vi "Configuration.vi"(0 "App Path":path=path "C:/Users/gtetil/Documents/Projects/DAQ Rack/Source", 5 "Config Path":path, 7 "Cal Base Path":path) -> (6 "Config Path OUT":path)   [LabVIEW 2019]
uses:
  Type Defs and Controls/Sensor List Cluster.ctl
  Type Defs and Controls/Channel Config Screen.ctl
  Type Defs and Controls/Log File Type.ctl
  Type Defs and Controls/Registered System.ctl
  Type Defs and Controls/System Type.ctl
  Type Defs and Controls/Sensor Config.ctl
  Type Defs and Controls/DAQ Settings.ctl
  Type Defs and Controls/Trigger Stop Method.ctl
  Type Defs and Controls/Channel Config.ctl
  Type Defs and Controls/Header.ctl
  Type Defs and Controls/Graph Settings Type Def.ctl
  Type Defs and Controls/Test Limits.ctl
  Type Defs and Controls/All Part Info.ctl
  Type Defs and Controls/Part Info.ctl
  <vilib>/Utility/config.llb/Write Key (Path).vi
  <vilib>/Utility/config.llb/NI_LVConfig.lvlib
panel:
  in  "TCP Stream Ref":refnum<vi>
  in  "System":T1={"System Type"=enum."DAQ Cart", "Serial Number"=0, "ID"="", "Cal File?"=FALSE}
  in  "Log File Type":T3
  in  "Part Config":bool
  in  "Limit:":dbl caption="Mb"
  in  "Hide Trig Ch":bool
  in  "Hide Trig Val":bool
  in  "Hide Trig Samples":bool
  in  "Hide Trig Stop":bool
  in  "Hide Trig Int":bool
  in  "Hide Pretrig Smpls":bool
  in  "Save Mode":T4(ring)
  in  "Sample Min":bool
  in  "Sample Sec":bool
  out "Changes Latch":bool
  out "Changes?":bool
  in  "Revert":bool
  out "Config Name":string
  in  "debug":bool
  in  "Delete Sensor":bool
  in  "Add Sensor":bool
  in  "Save As":bool
  in  "Save":bool
  in  "Open":bool
  in  "Calling VI Ref":refnum<vi>
  in  "Auto Save":bool=TRUE
  in  "Trigger Stop Method":T5(ring)
  in  "Hours":bool
  in  "Minutes":bool
  in  "Trigger Type":T6(ring)
  in  "Header Table":string[][](table)=[[""], [""], [""], [""], [""], [""]]
  in  "Sensors":T7=[{"Channel"="9221_AI-00", "Description"="", "Acquire"=FALSE, "Sensor"="None Selected", "Chg Sensor"=FALSE, "Cal Date"="---------", "Offset"=0.0, "Span"=0.0, "Cal"=FALSE, "Test Limits"=FALSE, "Type"="0-60 VDC", "Data Index"=0}, {"Channel"="9221_AI-01", "Description"="", "Acquire"=FALSE, "Sensor"="None Selected", "Chg Sensor"=FALSE, "Cal Date"="---------", "Offset"=0.0, "Span"=0.0, "Cal"=FALSE, "Test Limits"=FALSE, "Type"="0-60 VDC", "Data Index"=1}, {"Channel"="9221_AI-02", "Description"="", "Acquire"=FALSE, "Sensor"="None Selected", "Chg Sensor"=FALSE, "Cal Date"="---------", "Offset"=0.0, "Span"=0.0, "Cal"=FALSE, "Test Limits"=FALSE, "Type"="0-60 VDC", "Data Index"=2}, {"Channel"="9221_AI-03", "Description"="", "Acquire"=FALSE, "Sensor"="None Selected", "Chg Sensor"=FALSE, "Cal Date"="---------", "Offset"=0.0, "Span"=0.0, "Cal"=FALSE, "Test Limits"=FALSE, "Type"="0-60 VDC", "Data Index"=3}, {"Channel"="9221_AI-04", "Description"="", "Acquire"=FALSE, "Sensor"="None Selected", "Chg Sensor"=FALSE, "Cal Date"="---------", "Offset"=0.0, "Span"=0.0, "Cal"=FALSE, "Test Limits"=FALSE, "Type"="0-60 VDC", "Data Index"=4}, {"Channel"="9221_AI-05", "Description"="", "Acquire"=FALSE, "Sensor"="None Selected", "Chg Sensor"=FALSE, "Cal Date"="---------", "Offset"=0.0, "Span"=0.0, "Cal"=FALSE, "Test Limits"=FALSE, "Type"="0-60 VDC", "Data Index"=5}, {"Channel"="9221_AI-06", "Description"="", "Acquire"=FALSE, "Sensor"="None Selected", "Chg Sensor"=FALSE, "Cal Date"="---------", "Offset"=0.0, "Span"=0.0, "Cal"=FALSE, "Test Limits"=FALSE, "Type"="0-60 VDC", "Data Index"=6}, {"Channel"="9221_AI-07", "Description"="", "Acquire"=FALSE, "Sensor"="None Selected", "Chg Sensor"=FALSE, "Cal Date"="---------", "Offset"=0.0, "Span"=0.0, "Cal"=FALSE, "Test Limits"=FALSE, "Type"="0-60 VDC", "Data Index"=7}, {"Channel"="9205_AI-00", "Description"="", "Acquire"=FALSE, "Sensor"="None Selected", "Chg Sensor"=FALSE, "Cal Date"="---------", "Offset"=0.0, "Span"=0.0, "Cal"=FALSE, "Test Limits"=FALSE, "Type"="0-10 VDC", "Data Index"=8}, {"Channel"="9205_AI-01", "Description"="", "Acquire"=FALSE, "Sensor"="None Selected", "Chg Sensor"=FALSE, "Cal Date"="---------", "Offset"=0.0, "Span"=0.0, "Cal"=FALSE, "Test Limits"=FALSE, "Type"="0-10 VDC", "Data Index"=9}, {"Channel"="9205_AI-02", "Description"="", "Acquire"=FALSE, "Sensor"="None Selected", "Chg Sensor"=FALSE, "Cal Date"="---------", "Offset"=0.0, "Span"=0.0, "Cal"=FALSE, "Test Limits"=FALSE, "Type"="0-10 VDC", "Data Index"=10}, {"Channel"="9205_AI-03", "Description"="", "Acquire"=FALSE, "Sensor"="None Selected", "Chg Sensor"=FALSE, "Cal Date"="---------", "Offset"=0.0, "Span"=0.0, "Cal"=FALSE, "Test Limits"=FALSE, "Type"="0-10 VDC", "Data Index"=11}, {"Channel"="9205_AI-04", "Description"="", "Acquire"=FALSE, "Sensor"="None Selected", "Chg Sensor"=FALSE, "Cal Date"="---------", "Offset"=0.0, "Span"=0.0, "Cal"=FALSE, "Test Limits"=FALSE, "Type"="0-10 VDC", "Data Index"=12}, {"Channel"="9205_AI-05", "Description"="", "Acquire"=FALSE, "Sensor"="None Selected", "Chg Sensor"=FALSE, "Cal Date"="---------", "Offset"=0.0, "Span"=0.0, "Cal"=FALSE, "Test Limits"=FALSE, "Type"="0-10 VDC", "Data Index"=13}, {"Channel"="9205_AI-06", "Description"="", "Acquire"=FALSE, "Sensor"="None Selected", "Chg Sensor"=FALSE, "Cal Date"="---------", "Offset"=0.0, "Span"=0.0, "Cal"=FALSE, "Test Limits"=FALSE, "Type"="0-10 VDC", "Data Index"=14}, {"Channel"="9205_AI-07", "Description"="", "Acquire"=FALSE, "Sensor"="None Selected", "Chg Sensor"=FALSE, "Cal Date"="---------", "Offset"=0.0, "Span"=0.0, "Cal"=FALSE, "Test Limits"=FALSE, "Type"="0-10 VDC", "Data Index"=15}, {"Channel"="9208_AI-00", "Description"="", "Acquire"=FALSE, "Sensor"="None Selected", "Chg Sensor"=FALSE, "Cal Date"="---------", "Offset"=0.0, "Span"=0.0, "Cal"=FALSE, "Test Limits"=FALSE, "Type"="0-20 mA", "Data Index"=16}, {"Channel"="9208_AI-01", "Description"="", "Acquire"=FALSE, "Sensor"="None Selected", "Chg Sensor"=FALSE, "Cal Date"="---------", "Offset"=0.0, "Span"=0.0, "Cal"=FALSE, "Test Limits"=FALSE, "Type"="0-20 mA", "Data Index"=17}, {"Channel"="9208_AI-02", "Description"="", "Acquire"=FALSE, "Sensor"="None Selected", "Chg Sensor"=FALSE, "Cal Date"="---------", "Offset"=0.0, "Span"=0.0, "Cal"=FALSE, "Test Limits"=FALSE, "Type"="0-20 mA", "Data Index"=18}, {"Channel"="9208_AI-03", "Description"="", "Acquire"=FALSE, "Sensor"="None Selected", "Chg Sensor"=FALSE, "Cal Date"="---------", "Offset"=0.0, "Span"=0.0, "Cal"=FALSE, "Test Limits"=FALSE, "Type"="0-20 mA", "Data Index"=19}, {"Channel"="9208_AI-04", "Description"="", "Acquire"=FALSE, "Sensor"="None Selected", "Chg Sensor"=FALSE, "Cal Date"="---------", "Offset"=0.0, "Span"=0.0, "Cal"=FALSE, "Test Limits"=FALSE, "Type"="0-20 mA", "Data Index"=20}, {"Channel"="9208_AI-05", "Description"="", "Acquire"=FALSE, "Sensor"="None Selected", "Chg Sensor"=FALSE, "Cal Date"="---------", "Offset"=0.0, "Span"=0.0, "Cal"=FALSE, "Test Limits"=FALSE, "Type"="0-20 mA", "Data Index"=21}, {"Channel"="9208_AI-06", "Description"="", "Acquire"=FALSE, "Sensor"="None Selected", "Chg Sensor"=FALSE, "Cal Date"="---------", "Offset"=0.0, "Span"=0.0, "Cal"=FALSE, "Test Limits"=FALSE, "Type"="0-20 mA", "Data Index"=22}, {"Channel"="9208_AI-07", "Description"="", "Acquire"=FALSE, "Sensor"="None Selected", "Chg Sensor"=FALSE, "Cal Date"="---------", "Offset"=0.0, "Span"=0.0, "Cal"=FALSE, "Test Limits"=FALSE, "Type"="0-20 mA", "Data Index"=23}, {"Channel"="9211_TC-00", "Description"="", "Acquire"=FALSE, "Sensor"="None Selected", "Chg Sensor"=FALSE, "Cal Date"="---------", "Offset"=0.0, "Span"=0.0, "Cal"=FALSE, "Test Limits"=FALSE, "Type"="T-Type", "Data Index"=24}, {"Channel"="9211_TC-01", "Description"="", "Acquire"=FALSE, "Sensor"="None Selected", "Chg Sensor"=FALSE, "Cal Date"="---------", "Offset"=0.0, "Span"=0.0, "Cal"=FALSE, "Test Limits"=FALSE, "Type"="T-Type", "Data Index"=25}, {"Channel"="9211_TC-02", "Description"="", "Acquire"=FALSE, "Sensor"="None Selected", "Chg Sensor"=FALSE, "Cal Date"="---------", "Offset"=0.0, "Span"=0.0, "Cal"=FALSE, "Test Limits"=FALSE, "Type"="T-Type", "Data Index"=26}, {"Channel"="9211_TC-03", "Description"="", "Acquire"=FALSE, "Sensor"="None Selected", "Chg Sensor"=FALSE, "Cal Date"="---------", "Offset"=0.0, "Span"=0.0, "Cal"=FALSE, "Test Limits"=FALSE, "Type"="T-Type", "Data Index"=27}]
  in  "DAQ Table":string[][](table)=[[""], ["AI-00"], ["0.000"], ["0"], ["0"], ["0.000"], [""], ["100"]]
  # "samples /"
  # "Channel"
  # "Type"
  # "Acquire"
  # "Name"
  # "Sensor"
  # "Cal Date"
  # "Zero"
  # "Span"
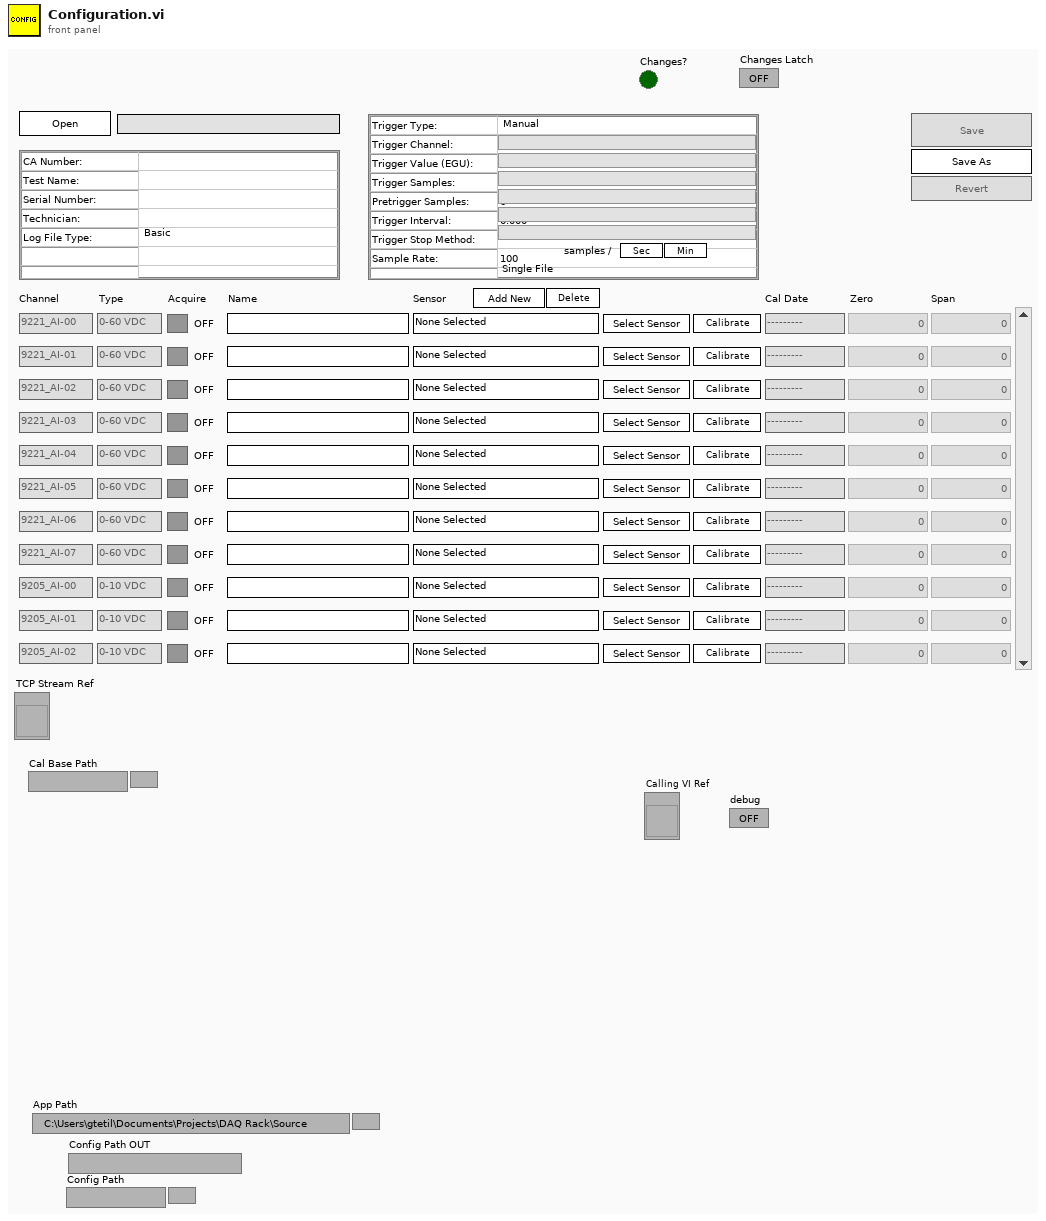
[diagram p1: front panel]
types:
  T1 = typedef "Registered System.ctl" = cluster{"System Type":T2, "Serial Number":u32, "ID":string, "Cal File?":bool}
  T2 = typedef "System Type.ctl" = enum16{"DAQ Rack", "DAQ Cart", "nx-5000", "unknown", "open"}
  T3 = typedef "Log File Type.ctl" = enum16{"Basic", "RTS"}
  T4 = enum16{"Single File", "Segmented Files", "New File at Midnight"}
  T5 = enum16{"Use Samples Value to Stop Trigger", "Use Threshold to Stop Trigger"}
  T6 = enum16{"Manual", "Timed", "Analog Rising", "Analog Falling"}
  T7 = typedef "Sensor List Cluster.ctl" = T8[]
  T8 = typedef "Channel Config Screen.ctl" = cluster{"Channel":string, "Description":string, "Acquire":bool, "Sensor":string, "Chg Sensor":bool, "Cal Date":string, "Offset":dbl, "Span":dbl, "Cal":bool, "Test Limits":bool, "Type":string, "Data Index":u32}
  T9 = typedef "Sensor Config.ctl" = cluster{"DAQ Settings":T10, "Channels":T12[], "Header":T13, "Graph Settings":T14, "Test Limits":T15[], "All Type Info":T16, "Save Mode":enum16{"Single File", "Segmented Files", "New File at Midnight"}}
  T10 = typedef "DAQ Settings.ctl" = cluster{"Trigger Type":enum16{"Manual", "Timed", "Analog Rising", "Analog Falling"}, "Trigger Samples":i32, "Pretrigger Samples":i32, "Trigger Interval":dbl, "Time Units":bool, "Auto Save":bool, "Sample Rate":dbl, "Select Analog":bool, "Trigger Value":dbl, "Trigger Stop Method":T11, "Rate Sec/Min":bool, "Save Mode":enum16{"Single File", "Segmented Files", "New File at Midnight"}, "File Size Limit":dbl, "Log File Type":T3, "Trigger Data Index":u32}
  T11 = typedef "Trigger Stop Method.ctl" = enum16{"Use Samples Value to Stop Trigger", "Use Threshold to Stop Trigger"}
  T12 = typedef "Channel Config.ctl" = cluster{"Channel":string, "Type":string, "Acquire":bool, "Name":string, "Sensor":string, "Data Index":u32}
  T13 = typedef "Header.ctl" = cluster{"TA Number":string, "Test Name":string, "Serial Number":string, "Technician":string}
  T14 = typedef "Graph Settings Type Def.ctl" = cluster{"Graph Labels":string[], u8[], i16[], u32[], u8[], u8[], u8[], u32[], u8[], u8[], u8[], dbl[], dbl[], "Graph Toggles":bool[], "Axis Toggles":bool[], "Graph Range":enum16{"1", "2", "3", "4", "5", "10", "15", "30", "60"}}
  T15 = typedef "Test Limits.ctl" = cluster{"Channel Acquired?":bool, "RMS?":bool, "Pk-Pk":bool, "Frequency":bool, "EU High Limit 1":dbl, "EU Low Limit 1":dbl, "EU High Limit 2":dbl, "EU Low Limit 2":dbl, "RMS High Limit":dbl, "RMS Low Limit":dbl, "Pk-Pk High Limit ":dbl, "Pk-Pk Low Limit":dbl, "Frequency High Limit":dbl, "Frequency Low Limit":dbl}
  T16 = typedef "All Part Info.ctl" = cluster{"Type Name":string, "Type Signal Names":string[], "# Signals":i32, "# Parts":i32, "Part Info":T17[]}[]
  T17 = typedef "Part Info.ctl" = cluster{"Part Number":string, "Channel Indexes":u16[], "Enabled?":bool}
  T18 = cluster{"Sensor Name":string, "Sensor Info":cluster{"Manufacturer":string, "Model":string, "Serial Number":string}, "Last Cal Info":cluster{"Last Calibration Date":dbl, "Calibrator":string, "Cal Duration":i32}, "Voltage Range":cluster{"High Limit":dbl, "Low Limit":dbl}, "EGU Range":cluster{"High Limit":dbl, "Low Limit":dbl}, "Units":string, "Calibration Type":enum16{"Calibrate Analog", "Compare Analog Calibration"}, "EGU List":dbl[], "Voltage List":dbl[], "Coefficients":dbl[], "Order":i32, "Algorithm":enum32{"SVD", "Givens", "Givens2", "Householder", "LU Decomposition", "Cholesky"}, "Max Error % of Full Scale":dbl, "Max Mean Squared Error":dbl, "Use Error %":bool, "Use MSE":bool, "Allow Manual Entry":bool, "Max Stability Error":dbl, "Max Error % of Reading":dbl, "Use Error % of Reading":bool}[]
  T19 = cluster{"Config Path":path, "Channel Select":i32, "Channel Display":T7, "App Path":path, "Config":T9, "Sensors":cluster{"Sensor Name":string, "Sensor Info":cluster{"Manufacturer":string, "Model":string, "Serial Number":string}, "Last Cal Info":cluster{"Last Calibration Date":dbl, "Calibrator":string, "Cal Duration":i32}, "Voltage Range":cluster{"High Limit":dbl, "Low Limit":dbl}, "EGU Range":cluster{"High Limit":dbl, "Low Limit":dbl}, "Units":string, "Calibration Type":enum16{"Calibrate Analog", "Compare Analog Calibration"}, "EGU List":dbl[], "Voltage List":dbl[], "Coefficients":dbl[], "Order":i32, "Algorithm":enum32{"SVD", "Givens", "Givens2", "Householder", "LU Decomposition", "Cholesky"}, "Max Error % of Full Scale":dbl, "Max Mean Squared Error":dbl, "Use Error %":bool, "Use MSE":bool, "Allow Manual Entry":bool, "Max Stability Error":dbl, "Max Error % of Reading":dbl, "Use Error % of Reading":bool}[], "Config Saved":T9, "config start path":path, "Cal Base Path":path, "Calling VI Ref":refnum<vi>, "debug":bool, "Changes?":bool, "Revert":bool, "DAQ Running":bool, "System":T1, "Load Prompt":bool, "App Config Path":path, "TCP Stream Ref":refnum<vi>}
  T20 = enum32{"Bad", "Idle", "Run top level", "Running"}
  T21 = enum8{"Enabled", "Disabled", "Disabled and Grayed Out"}
  T22 = typedef "eventvkey.ctl" = enum16{"ASCII", "Enter", "Return", "Shift", "Ctrl", "Alt", "Cmd", "Opt", "Caps", "NumLock", "Clear", "Break", "Up", "Down", "Left", "Right", "Insert", "Delete", "Home", "End", "PageUp", "PageDown", "Escape", "Help", "Pause", "ScrollLock", "F1", "F2", "F3", "F4", "F5", "F6", "F7", "F8", "F9", "F10", "F11", "F12", "F13", "F14", "F15", "F16", "F17", "F18", "F19", "F20", "F21", "F22", "F23", "F24", "Play", "VolumeUp", "VolumeDown", "Mute", "Two Byte Char"}
  T23 = typedef "LVRowAndColumnTypeDef.ctl" = cluster{"Row":i32, "Column":i32}
  T24 = cluster{"Header Table[0]":string, "Header Table[1]":string, "Header Table[2]":string, "Header Table[3]":string}
  T25 = typedef "LVPoint32TypeDef.ctl" = cluster{"Horizontal":i32, "Vertical":i32}
  T26 = cluster{"Sensor Name":string, "Sensor Info":cluster{"Manufacturer":string, "Model":string, "Serial Number":string}, "Last Cal Info":cluster{"Last Calibration Date":dbl, "Calibrator":string, "Cal Duration":i32}, "Voltage Range":cluster{"High Limit":dbl, "Low Limit":dbl}, "EGU Range":cluster{"High Limit":dbl, "Low Limit":dbl}, "Units":string, "Calibration Type":enum16{"Calibrate Analog", "Compare Analog Calibration"}, "EGU List":dbl[], "Voltage List":dbl[], "Coefficients":dbl[], "Order":i32, "Algorithm":enum32{"SVD", "Givens", "Givens2", "Householder", "LU Decomposition", "Cholesky"}, "Max Error % of Full Scale":dbl, "Max Mean Squared Error":dbl, "Use Error %":bool, "Use MSE":bool, "Allow Manual Entry":bool, "Max Stability Error":dbl, "Max Error % of Reading":dbl, "Use Error % of Reading":bool}
  T27 = typedef "NI_LVConfig.lvlib/Config Data RefNum.ctl" = refnum<k1>
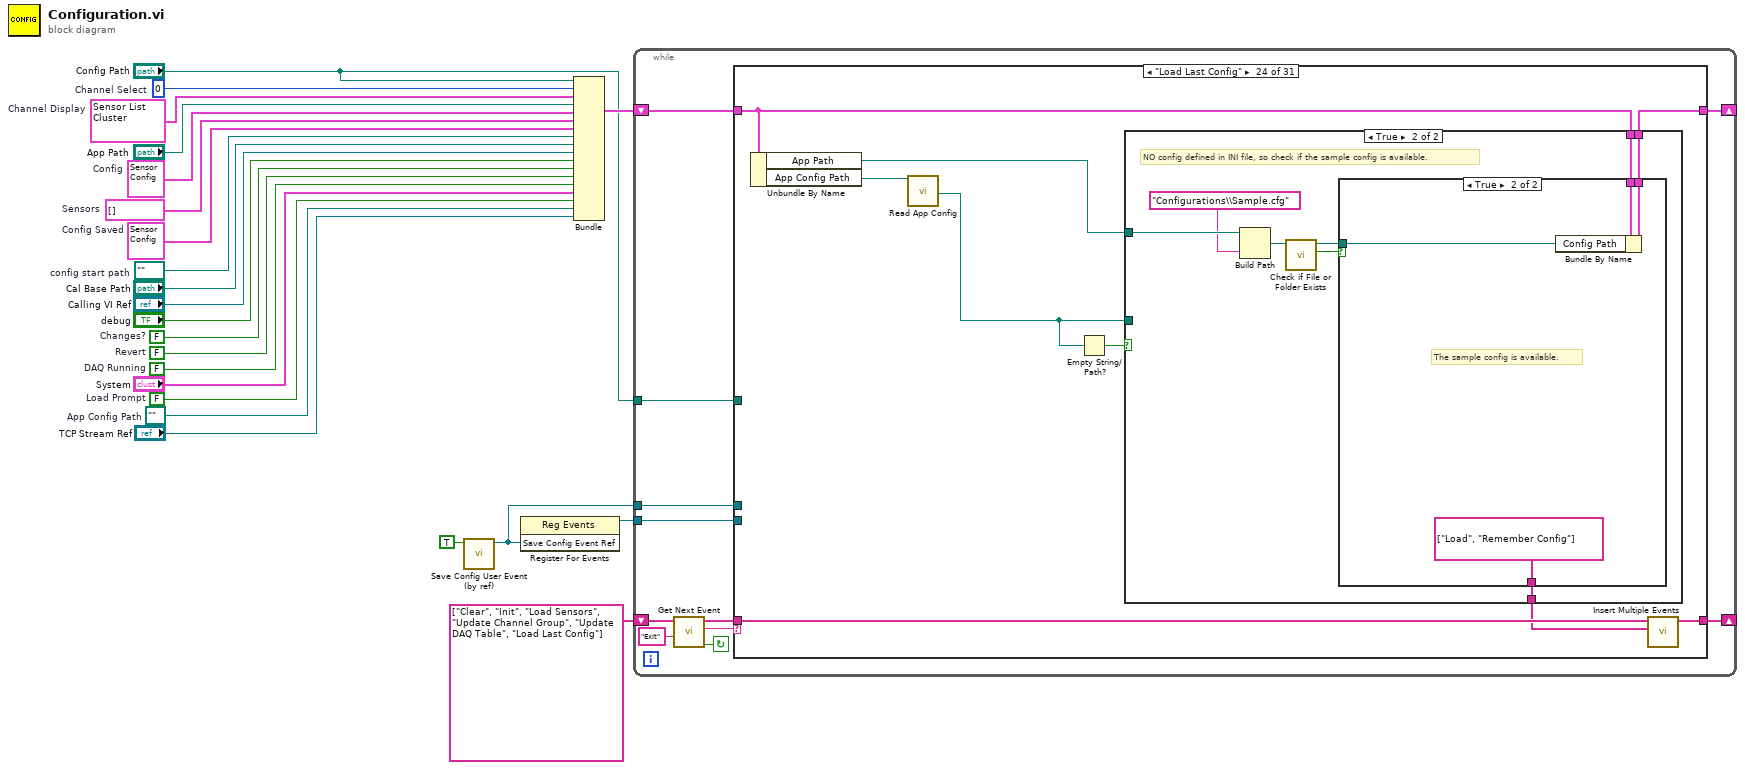
[diagram p0: block diagram]
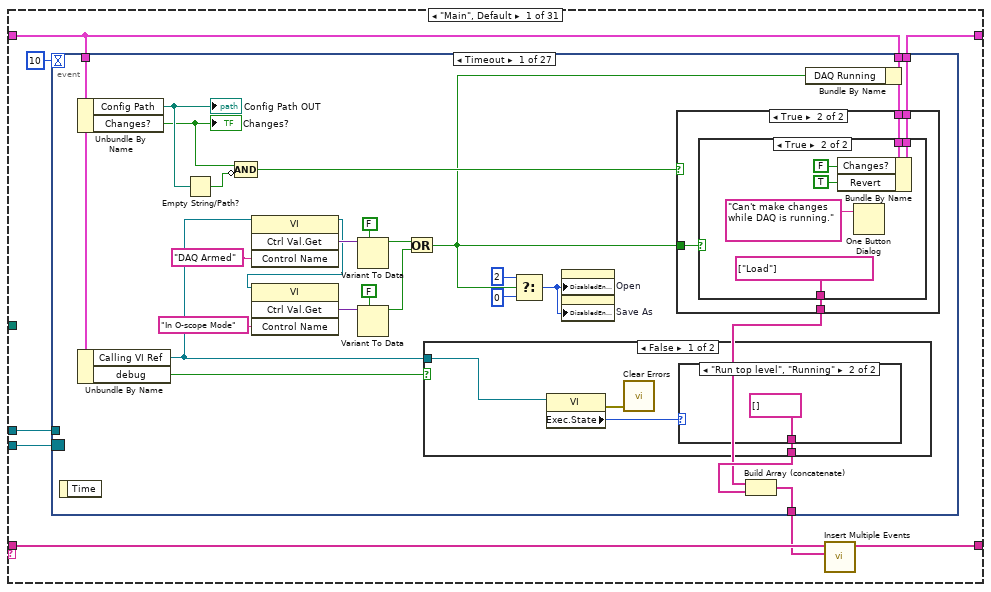
[diagram p2: hidden frame]
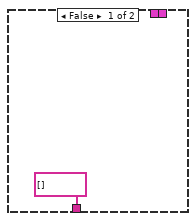
[diagram p3: hidden frame]
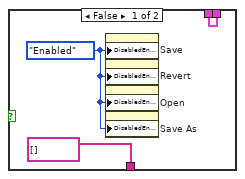
[diagram p4: hidden frame]
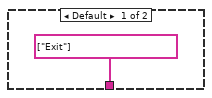
[diagram p5: hidden frame]
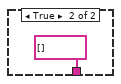
[diagram p6: hidden frame]
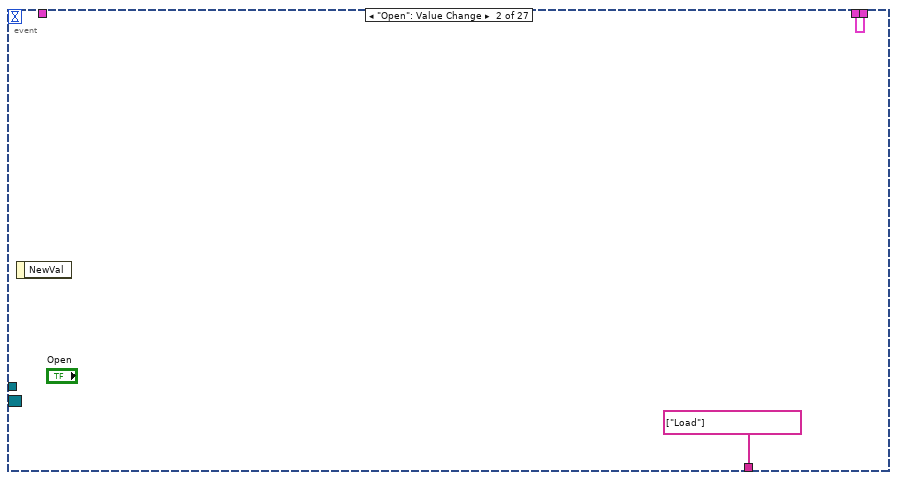
[diagram p7: hidden frame]
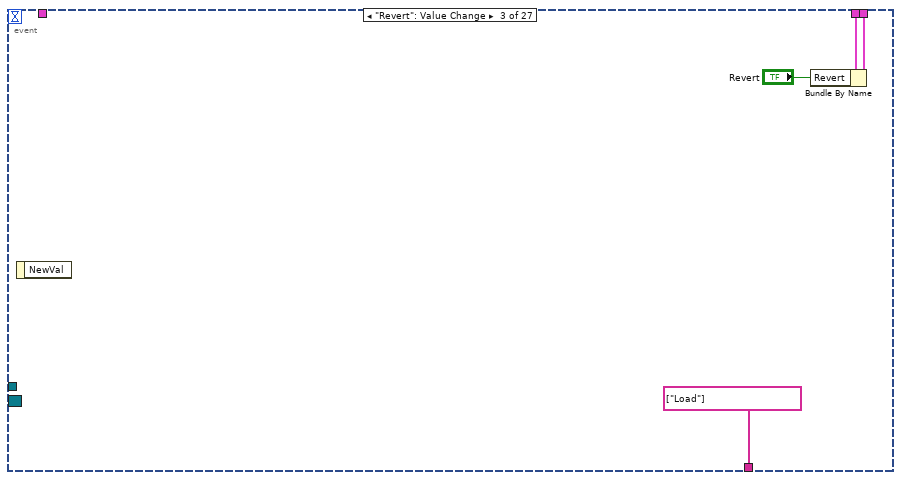
[diagram p8: hidden frame]
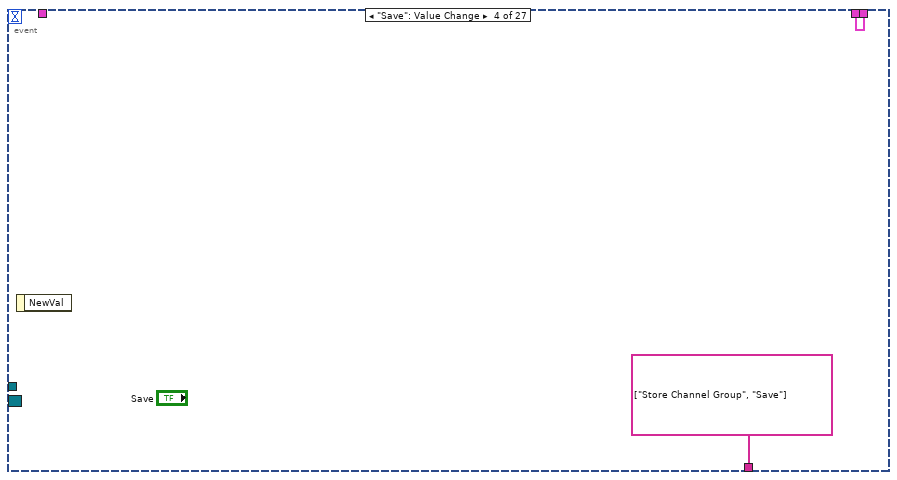
[diagram p9: hidden frame]
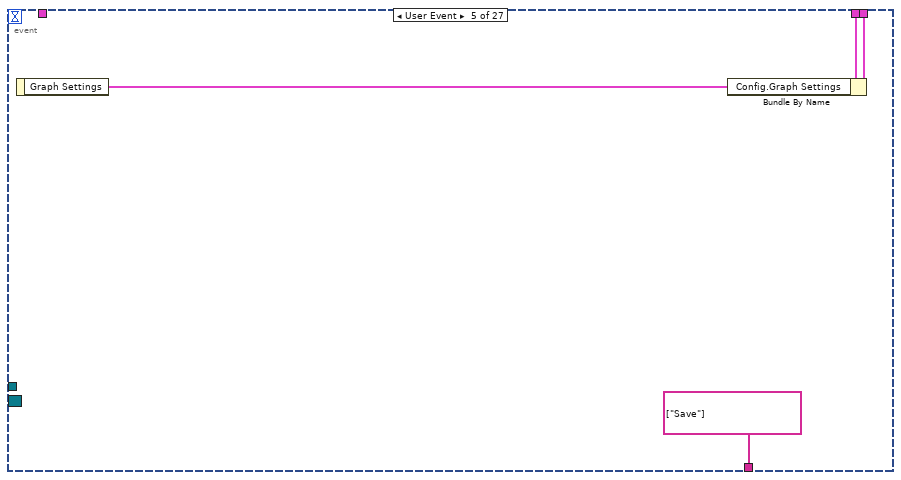
[diagram p10: hidden frame]
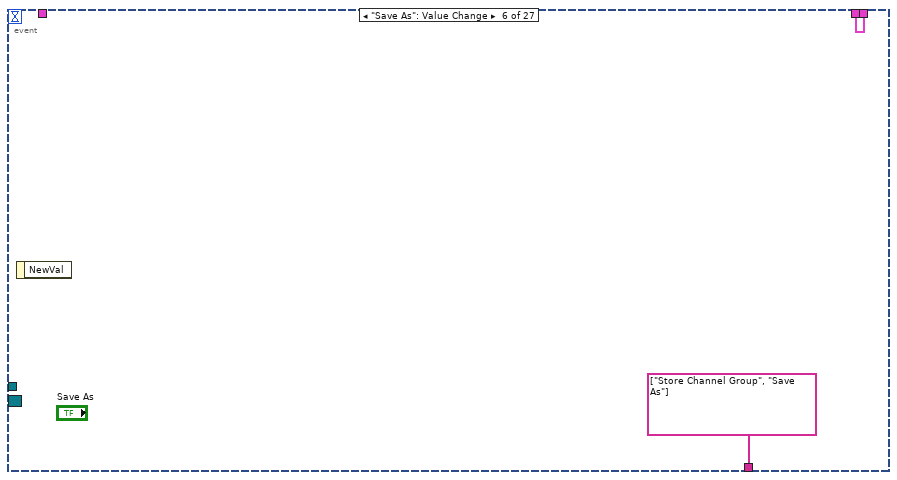
[diagram p11: hidden frame]
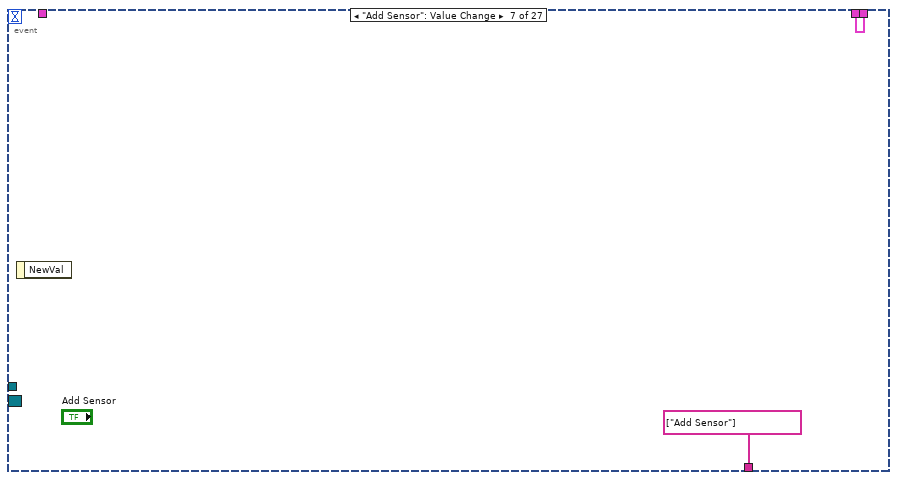
[diagram p12: hidden frame]
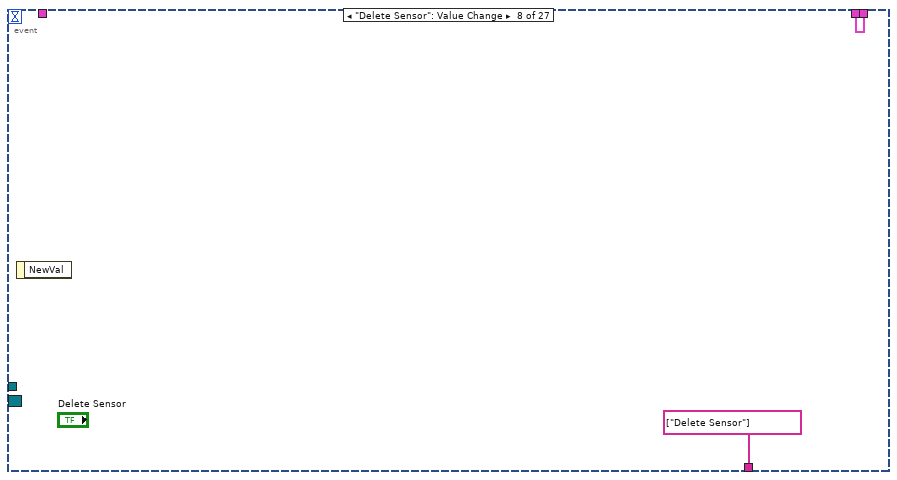
[diagram p13: hidden frame]
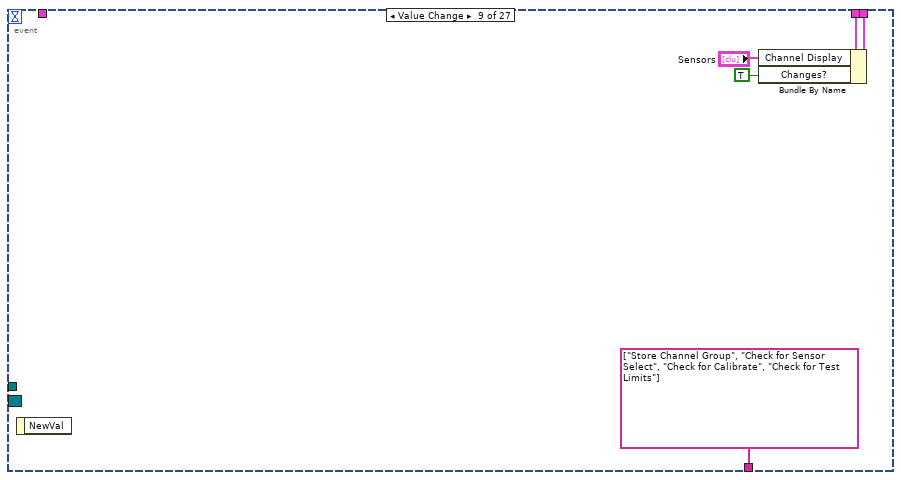
[diagram p14: hidden frame]
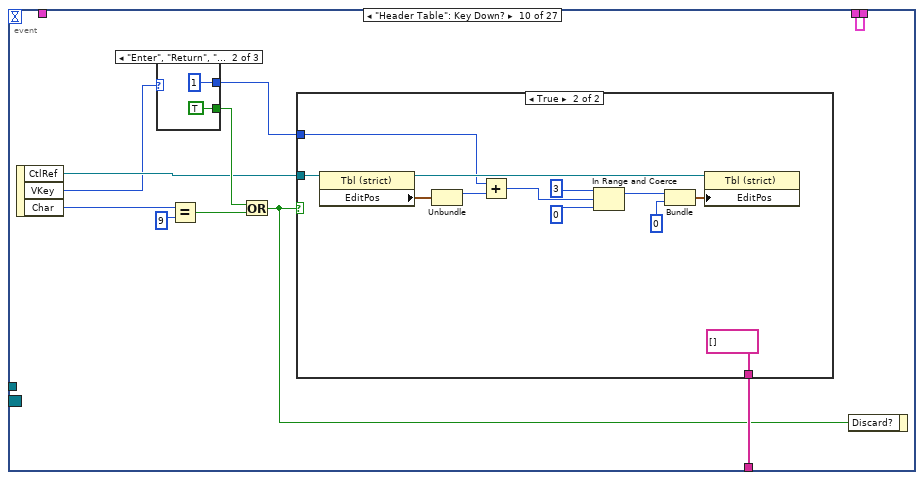
[diagram p15: hidden frame]
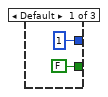
[diagram p16: hidden frame]
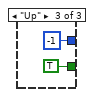
[diagram p17: hidden frame]
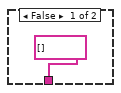
[diagram p18: hidden frame]
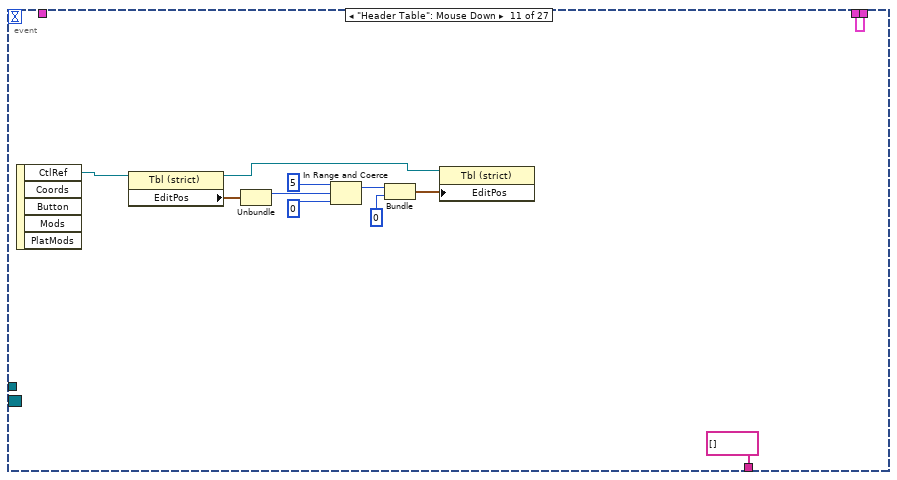
[diagram p19: hidden frame]
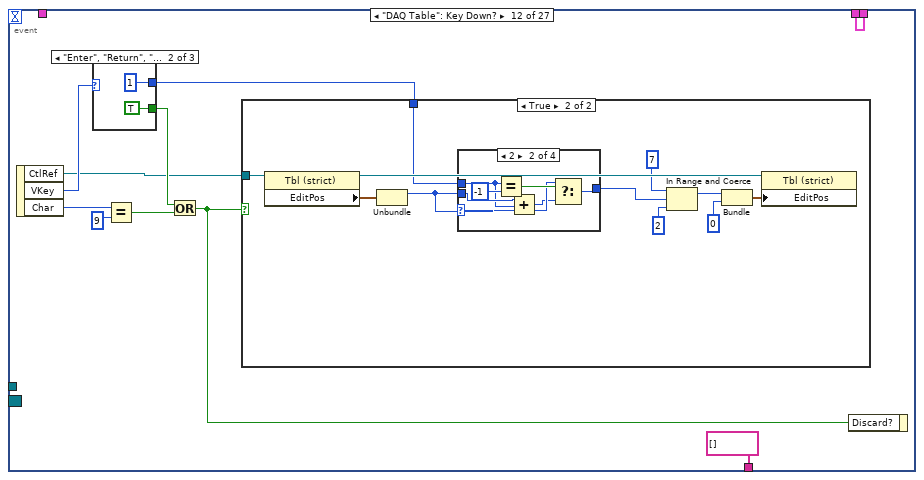
[diagram p20: hidden frame]
diagram:
  w2 = path ""  # App Config Path
  w4 = FALSE  # Load Prompt
  w6 = FALSE  # DAQ Running
  w10 = FALSE  # Revert
  w11 = FALSE  # Changes?
  w15 = path ""  # config start path
  w17 = T9 {"DAQ Settings"={"Trigger Type"=enum."Manual", "Trigger Samples"=0, "Pretrigger Samples"=0, "Trigger Interval"=0.0, "Time Units"=FALSE, "Auto Save"=FALSE, "Sample Rate"=0.0, "Select Analog"=FALSE, "Trigger Value"=0.0, "Trigger Stop Method"=enum."Use Samples Value to Stop Trigger", "Rate Sec/Min"=FALSE, "Save Mode"=enum."Single File", "File Size Limit"=0.0, "Log File Type"=enum."Basic", "Trigger Data Index"=0}, "Channels"=[], "Header"={"TA Number"="", "Test Name"="", "Serial Number"="", "Technician"=""}, "Graph Settings"={"Graph Labels"=[], [], [], [], [], [], [], [], [], [], [], [], [], "Graph Toggles"=[], "Axis Toggles"=[], "Graph Range"=enum."1"}, "Test Limits"=[], "All Type Info"=[], "Save Mode"=enum."Single File"}  # Config Saved
  w5 = T9 {"DAQ Settings"={"Trigger Type"=enum."Manual", "Trigger Samples"=0, "Pretrigger Samples"=0, "Trigger Interval"=0.0, "Time Units"=FALSE, "Auto Save"=FALSE, "Sample Rate"=0.0, "Select Analog"=FALSE, "Trigger Value"=0.0, "Trigger Stop Method"=enum."Use Samples Value to Stop Trigger", "Rate Sec/Min"=FALSE, "Save Mode"=enum."Single File", "File Size Limit"=0.0, "Log File Type"=enum."Basic", "Trigger Data Index"=0}, "Channels"=[], "Header"={"TA Number"="", "Test Name"="", "Serial Number"="", "Technician"=""}, "Graph Settings"={"Graph Labels"=[], [], [], [], [], [], [], [], [], [], [], [], [], "Graph Toggles"=[], "Axis Toggles"=[], "Graph Range"=enum."1"}, "Test Limits"=[], "All Type Info"=[], "Save Mode"=enum."Single File"}  # Config
  w18 = T18 []  # Sensors
  w19 = 0  # Channel Select
  w20 = T7 [{"Channel"="", "Description"="", "Acquire"=FALSE, "Sensor"="", "Chg Sensor"=FALSE, "Cal Date"="", "Offset"=0.0, "Span"=0.0, "Cal"=FALSE, "Test Limits"=FALSE, "Type"="", "Data Index"=0}, {"Channel"="", "Description"="", "Acquire"=FALSE, "Sensor"="", "Chg Sensor"=FALSE, "Cal Date"="", "Offset"=0.0, "Span"=0.0, "Cal"=FALSE, "Test Limits"=FALSE, "Type"="", "Data Index"=0}, {"Channel"="", "Description"="", "Acquire"=FALSE, "Sensor"="", "Chg Sensor"=FALSE, "Cal Date"="", "Offset"=0.0, "Span"=0.0, "Cal"=FALSE, "Test Limits"=FALSE, "Type"="", "Data Index"=0}, {"Channel"="", "Description"="", "Acquire"=FALSE, "Sensor"="", "Chg Sensor"=FALSE, "Cal Date"="", "Offset"=0.0, "Span"=0.0, "Cal"=FALSE, "Test Limits"=FALSE, "Type"="", "Data Index"=0}, {"Channel"="", "Description"="", "Acquire"=FALSE, "Sensor"="", "Chg Sensor"=FALSE, "Cal Date"="", "Offset"=0.0, "Span"=0.0, "Cal"=FALSE, "Test Limits"=FALSE, "Type"="", "Data Index"=0}, {"Channel"="", "Description"="", "Acquire"=FALSE, "Sensor"="", "Chg Sensor"=FALSE, "Cal Date"="", "Offset"=0.0, "Span"=0.0, "Cal"=FALSE, "Test Limits"=FALSE, "Type"="", "Data Index"=0}, {"Channel"="", "Description"="", "Acquire"=FALSE, "Sensor"="", "Chg Sensor"=FALSE, "Cal Date"="", "Offset"=0.0, "Span"=0.0, "Cal"=FALSE, "Test Limits"=FALSE, "Type"="", "Data Index"=0}, {"Channel"="", "Description"="", "Acquire"=FALSE, "Sensor"="", "Chg Sensor"=FALSE, "Cal Date"="", "Offset"=0.0, "Span"=0.0, "Cal"=FALSE, "Test Limits"=FALSE, "Type"="", "Data Index"=0}, {"Channel"="", "Description"="", "Acquire"=FALSE, "Sensor"="", "Chg Sensor"=FALSE, "Cal Date"="", "Offset"=0.0, "Span"=0.0, "Cal"=FALSE, "Test Limits"=FALSE, "Type"="", "Data Index"=0}, {"Channel"="", "Description"="", "Acquire"=FALSE, "Sensor"="", "Chg Sensor"=FALSE, "Cal Date"="", "Offset"=0.0, "Span"=0.0, "Cal"=FALSE, "Test Limits"=FALSE, "Type"="", "Data Index"=0}, {"Channel"="", "Description"="", "Acquire"=FALSE, "Sensor"="", "Chg Sensor"=FALSE, "Cal Date"="", "Offset"=0.0, "Span"=0.0, "Cal"=FALSE, "Test Limits"=FALSE, "Type"="", "Data Index"=0}, {"Channel"="", "Description"="", "Acquire"=FALSE, "Sensor"="", "Chg Sensor"=FALSE, "Cal Date"="", "Offset"=0.0, "Span"=0.0, "Cal"=FALSE, "Test Limits"=FALSE, "Type"="", "Data Index"=0}, {"Channel"="", "Description"="", "Acquire"=FALSE, "Sensor"="", "Chg Sensor"=FALSE, "Cal Date"="", "Offset"=0.0, "Span"=0.0, "Cal"=FALSE, "Test Limits"=FALSE, "Type"="", "Data Index"=0}, {"Channel"="", "Description"="", "Acquire"=FALSE, "Sensor"="", "Chg Sensor"=FALSE, "Cal Date"="", "Offset"=0.0, "Span"=0.0, "Cal"=FALSE, "Test Limits"=FALSE, "Type"="", "Data Index"=0}, {"Channel"="", "Description"="", "Acquire"=FALSE, "Sensor"="", "Chg Sensor"=FALSE, "Cal Date"="", "Offset"=0.0, "Span"=0.0, "Cal"=FALSE, "Test Limits"=FALSE, "Type"="", "Data Index"=0}, {"Channel"="", "Description"="", "Acquire"=FALSE, "Sensor"="", "Chg Sensor"=FALSE, "Cal Date"="", "Offset"=0.0, "Span"=0.0, "Cal"=FALSE, "Test Limits"=FALSE, "Type"="", "Data Index"=0}, {"Channel"="", "Description"="", "Acquire"=FALSE, "Sensor"="", "Chg Sensor"=FALSE, "Cal Date"="", "Offset"=0.0, "Span"=0.0, "Cal"=FALSE, "Test Limits"=FALSE, "Type"="", "Data Index"=0}, {"Channel"="", "Description"="", "Acquire"=FALSE, "Sensor"="", "Chg Sensor"=FALSE, "Cal Date"="", "Offset"=0.0, "Span"=0.0, "Cal"=FALSE, "Test Limits"=FALSE, "Type"="", "Data Index"=0}, {"Channel"="", "Description"="", "Acquire"=FALSE, "Sensor"="", "Chg Sensor"=FALSE, "Cal Date"="", "Offset"=0.0, "Span"=0.0, "Cal"=FALSE, "Test Limits"=FALSE, "Type"="", "Data Index"=0}, {"Channel"="", "Description"="", "Acquire"=FALSE, "Sensor"="", "Chg Sensor"=FALSE, "Cal Date"="", "Offset"=0.0, "Span"=0.0, "Cal"=FALSE, "Test Limits"=FALSE, "Type"="", "Data Index"=0}, {"Channel"="", "Description"="", "Acquire"=FALSE, "Sensor"="", "Chg Sensor"=FALSE, "Cal Date"="", "Offset"=0.0, "Span"=0.0, "Cal"=FALSE, "Test Limits"=FALSE, "Type"="", "Data Index"=0}, {"Channel"="", "Description"="", "Acquire"=FALSE, "Sensor"="", "Chg Sensor"=FALSE, "Cal Date"="", "Offset"=0.0, "Span"=0.0, "Cal"=FALSE, "Test Limits"=FALSE, "Type"="", "Data Index"=0}, {"Channel"="", "Description"="", "Acquire"=FALSE, "Sensor"="", "Chg Sensor"=FALSE, "Cal Date"="", "Offset"=0.0, "Span"=0.0, "Cal"=FALSE, "Test Limits"=FALSE, "Type"="", "Data Index"=0}, {"Channel"="", "Description"="", "Acquire"=FALSE, "Sensor"="", "Chg Sensor"=FALSE, "Cal Date"="", "Offset"=0.0, "Span"=0.0, "Cal"=FALSE, "Test Limits"=FALSE, "Type"="", "Data Index"=0}, {"Channel"="", "Description"="", "Acquire"=FALSE, "Sensor"="", "Chg Sensor"=FALSE, "Cal Date"="", "Offset"=0.0, "Span"=0.0, "Cal"=FALSE, "Test Limits"=FALSE, "Type"="", "Data Index"=0}, {"Channel"="", "Description"="", "Acquire"=FALSE, "Sensor"="", "Chg Sensor"=FALSE, "Cal Date"="", "Offset"=0.0, "Span"=0.0, "Cal"=FALSE, "Test Limits"=FALSE, "Type"="", "Data Index"=0}, {"Channel"="", "Description"="", "Acquire"=FALSE, "Sensor"="", "Chg Sensor"=FALSE, "Cal Date"="", "Offset"=0.0, "Span"=0.0, "Cal"=FALSE, "Test Limits"=FALSE, "Type"="", "Data Index"=0}, {"Channel"="", "Description"="", "Acquire"=FALSE, "Sensor"="", "Chg Sensor"=FALSE, "Cal Date"="", "Offset"=0.0, "Span"=0.0, "Cal"=FALSE, "Test Limits"=FALSE, "Type"="", "Data Index"=0}, {"Channel"="", "Description"="", "Acquire"=FALSE, "Sensor"="", "Chg Sensor"=FALSE, "Cal Date"="", "Offset"=0.0, "Span"=0.0, "Cal"=FALSE, "Test Limits"=FALSE, "Type"="", "Data Index"=0}, {"Channel"="", "Description"="", "Acquire"=FALSE, "Sensor"="", "Chg Sensor"=FALSE, "Cal Date"="", "Offset"=0.0, "Span"=0.0, "Cal"=FALSE, "Test Limits"=FALSE, "Type"="", "Data Index"=0}, {"Channel"="", "Description"="", "Acquire"=FALSE, "Sensor"="", "Chg Sensor"=FALSE, "Cal Date"="", "Offset"=0.0, "Span"=0.0, "Cal"=FALSE, "Test Limits"=FALSE, "Type"="", "Data Index"=0}, {"Channel"="", "Description"="", "Acquire"=FALSE, "Sensor"="", "Chg Sensor"=FALSE, "Cal Date"="", "Offset"=0.0, "Span"=0.0, "Cal"=FALSE, "Test Limits"=FALSE, "Type"="", "Data Index"=0}, {"Channel"="", "Description"="", "Acquire"=FALSE, "Sensor"="", "Chg Sensor"=FALSE, "Cal Date"="", "Offset"=0.0, "Span"=0.0, "Cal"=FALSE, "Test Limits"=FALSE, "Type"="", "Data Index"=0}, {"Channel"="", "Description"="", "Acquire"=FALSE, "Sensor"="", "Chg Sensor"=FALSE, "Cal Date"="", "Offset"=0.0, "Span"=0.0, "Cal"=FALSE, "Test Limits"=FALSE, "Type"="", "Data Index"=0}, {"Channel"="", "Description"="", "Acquire"=FALSE, "Sensor"="", "Chg Sensor"=FALSE, "Cal Date"="", "Offset"=0.0, "Span"=0.0, "Cal"=FALSE, "Test Limits"=FALSE, "Type"="", "Data Index"=0}, {"Channel"="", "Description"="", "Acquire"=FALSE, "Sensor"="", "Chg Sensor"=FALSE, "Cal Date"="", "Offset"=0.0, "Span"=0.0, "Cal"=FALSE, "Test Limits"=FALSE, "Type"="", "Data Index"=0}, {"Channel"="", "Description"="", "Acquire"=FALSE, "Sensor"="", "Chg Sensor"=FALSE, "Cal Date"="", "Offset"=0.0, "Span"=0.0, "Cal"=FALSE, "Test Limits"=FALSE, "Type"="", "Data Index"=0}, {"Channel"="", "Description"="", "Acquire"=FALSE, "Sensor"="", "Chg Sensor"=FALSE, "Cal Date"="", "Offset"=0.0, "Span"=0.0, "Cal"=FALSE, "Test Limits"=FALSE, "Type"="", "Data Index"=0}, {"Channel"="", "Description"="", "Acquire"=FALSE, "Sensor"="", "Chg Sensor"=FALSE, "Cal Date"="", "Offset"=0.0, "Span"=0.0, "Cal"=FALSE, "Test Limits"=FALSE, "Type"="", "Data Index"=0}, {"Channel"="", "Description"="", "Acquire"=FALSE, "Sensor"="", "Chg Sensor"=FALSE, "Cal Date"="", "Offset"=0.0, "Span"=0.0, "Cal"=FALSE, "Test Limits"=FALSE, "Type"="", "Data Index"=0}, {"Channel"="", "Description"="", "Acquire"=FALSE, "Sensor"="", "Chg Sensor"=FALSE, "Cal Date"="", "Offset"=0.0, "Span"=0.0, "Cal"=FALSE, "Test Limits"=FALSE, "Type"="", "Data Index"=0}, {"Channel"="", "Description"="", "Acquire"=FALSE, "Sensor"="", "Chg Sensor"=FALSE, "Cal Date"="", "Offset"=0.0, "Span"=0.0, "Cal"=FALSE, "Test Limits"=FALSE, "Type"="", "Data Index"=0}, {"Channel"="", "Description"="", "Acquire"=FALSE, "Sensor"="", "Chg Sensor"=FALSE, "Cal Date"="", "Offset"=0.0, "Span"=0.0, "Cal"=FALSE, "Test Limits"=FALSE, "Type"="", "Data Index"=0}, {"Channel"="", "Description"="", "Acquire"=FALSE, "Sensor"="", "Chg Sensor"=FALSE, "Cal Date"="", "Offset"=0.0, "Span"=0.0, "Cal"=FALSE, "Test Limits"=FALSE, "Type"="", "Data Index"=0}, {"Channel"="", "Description"="", "Acquire"=FALSE, "Sensor"="", "Chg Sensor"=FALSE, "Cal Date"="", "Offset"=0.0, "Span"=0.0, "Cal"=FALSE, "Test Limits"=FALSE, "Type"="", "Data Index"=0}, {"Channel"="", "Description"="", "Acquire"=FALSE, "Sensor"="", "Chg Sensor"=FALSE, "Cal Date"="", "Offset"=0.0, "Span"=0.0, "Cal"=FALSE, "Test Limits"=FALSE, "Type"="", "Data Index"=0}, {"Channel"="", "Description"="", "Acquire"=FALSE, "Sensor"="", "Chg Sensor"=FALSE, "Cal Date"="", "Offset"=0.0, "Span"=0.0, "Cal"=FALSE, "Test Limits"=FALSE, "Type"="", "Data Index"=0}, {"Channel"="", "Description"="", "Acquire"=FALSE, "Sensor"="", "Chg Sensor"=FALSE, "Cal Date"="", "Offset"=0.0, "Span"=0.0, "Cal"=FALSE, "Test Limits"=FALSE, "Type"="", "Data Index"=0}, {"Channel"="", "Description"="", "Acquire"=FALSE, "Sensor"="", "Chg Sensor"=FALSE, "Cal Date"="", "Offset"=0.0, "Span"=0.0, "Cal"=FALSE, "Test Limits"=FALSE, "Type"="", "Data Index"=0}, {"Channel"="", "Description"="", "Acquire"=FALSE, "Sensor"="", "Chg Sensor"=FALSE, "Cal Date"="", "Offset"=0.0, "Span"=0.0, "Cal"=FALSE, "Test Limits"=FALSE, "Type"="", "Data Index"=0}, {"Channel"="", "Description"="", "Acquire"=FALSE, "Sensor"="", "Chg Sensor"=FALSE, "Cal Date"="", "Offset"=0.0, "Span"=0.0, "Cal"=FALSE, "Test Limits"=FALSE, "Type"="", "Data Index"=0}, {"Channel"="", "Description"="", "Acquire"=FALSE, "Sensor"="", "Chg Sensor"=FALSE, "Cal Date"="", "Offset"=0.0, "Span"=0.0, "Cal"=FALSE, "Test Limits"=FALSE, "Type"="", "Data Index"=0}, {"Channel"="", "Description"="", "Acquire"=FALSE, "Sensor"="", "Chg Sensor"=FALSE, "Cal Date"="", "Offset"=0.0, "Span"=0.0, "Cal"=FALSE, "Test Limits"=FALSE, "Type"="", "Data Index"=0}, {"Channel"="", "Description"="", "Acquire"=FALSE, "Sensor"="", "Chg Sensor"=FALSE, "Cal Date"="", "Offset"=0.0, "Span"=0.0, "Cal"=FALSE, "Test Limits"=FALSE, "Type"="", "Data Index"=0}, {"Channel"="", "Description"="", "Acquire"=FALSE, "Sensor"="", "Chg Sensor"=FALSE, "Cal Date"="", "Offset"=0.0, "Span"=0.0, "Cal"=FALSE, "Test Limits"=FALSE, "Type"="", "Data Index"=0}, {"Channel"="", "Description"="", "Acquire"=FALSE, "Sensor"="", "Chg Sensor"=FALSE, "Cal Date"="", "Offset"=0.0, "Span"=0.0, "Cal"=FALSE, "Test Limits"=FALSE, "Type"="", "Data Index"=0}, {"Channel"="", "Description"="", "Acquire"=FALSE, "Sensor"="", "Chg Sensor"=FALSE, "Cal Date"="", "Offset"=0.0, "Span"=0.0, "Cal"=FALSE, "Test Limits"=FALSE, "Type"="", "Data Index"=0}, {"Channel"="", "Description"="", "Acquire"=FALSE, "Sensor"="", "Chg Sensor"=FALSE, "Cal Date"="", "Offset"=0.0, "Span"=0.0, "Cal"=FALSE, "Test Limits"=FALSE, "Type"="", "Data Index"=0}, {"Channel"="", "Description"="", "Acquire"=FALSE, "Sensor"="", "Chg Sensor"=FALSE, "Cal Date"="", "Offset"=0.0, "Span"=0.0, "Cal"=FALSE, "Test Limits"=FALSE, "Type"="", "Data Index"=0}, {"Channel"="", "Description"="", "Acquire"=FALSE, "Sensor"="", "Chg Sensor"=FALSE, "Cal Date"="", "Offset"=0.0, "Span"=0.0, "Cal"=FALSE, "Test Limits"=FALSE, "Type"="", "Data Index"=0}, {"Channel"="", "Description"="", "Acquire"=FALSE, "Sensor"="", "Chg Sensor"=FALSE, "Cal Date"="", "Offset"=0.0, "Span"=0.0, "Cal"=FALSE, "Test Limits"=FALSE, "Type"="", "Data Index"=0}, {"Channel"="", "Description"="", "Acquire"=FALSE, "Sensor"="", "Chg Sensor"=FALSE, "Cal Date"="", "Offset"=0.0, "Span"=0.0, "Cal"=FALSE, "Test Limits"=FALSE, "Type"="", "Data Index"=0}, {"Channel"="", "Description"="", "Acquire"=FALSE, "Sensor"="", "Chg Sensor"=FALSE, "Cal Date"="", "Offset"=0.0, "Span"=0.0, "Cal"=FALSE, "Test Limits"=FALSE, "Type"="", "Data Index"=0}, {"Channel"="", "Description"="", "Acquire"=FALSE, "Sensor"="", "Chg Sensor"=FALSE, "Cal Date"="", "Offset"=0.0, "Span"=0.0, "Cal"=FALSE, "Test Limits"=FALSE, "Type"="", "Data Index"=0}, {"Channel"="", "Description"="", "Acquire"=FALSE, "Sensor"="", "Chg Sensor"=FALSE, "Cal Date"="", "Offset"=0.0, "Span"=0.0, "Cal"=FALSE, "Test Limits"=FALSE, "Type"="", "Data Index"=0}]  # Channel Display
  n1 = call "Save Config User Event (by ref).vi"("Register (F)"=TRUE) -> ("Save Config Event Ref"=w8:refnum<user-event>)  [unwired: 10 in]
  n2 = register-events(w8) -> (reference out=w9:refnum<event-registration>)  [unwired: 2 in, 1 out]
  n3 = Bundle("Config Path"="Config Path", "Channel Select"=w19, "Channel Display"=w20, "App Path"="App Path", "Config"=w5, "Sensors"=w18, "Config Saved"=w17, "config start path"=w15, "Cal Base Path"="Cal Base Path", "Calling VI Ref"="Calling VI Ref", "debug"="debug", "Changes?"=w11, "Revert"=w10, "DAQ Running"=w6, "System"="System", "Load Prompt"=w4, "App Config Path"=w2, "TCP Stream Ref"="TCP Stream Ref") -> (w22:T19)  [unwired: 1 in]
  n4 = while {
    shift-left: string[] ["Clear", "Init", "Load Sensors", "Update Channel Group", "Update DAQ Table", "Load Last Config"] ("event queue out") -> [w32]
    shift-right: [w28] -> _
    shift-left: w22 -> [w31]
    shift-right: [w30] -> _
    tunnel: "Config Path" -> [w26]
    tunnel: w9 -> [w25]
    tunnel: w8 -> [w24]
    stop <- w34 continue-if-true
    n5 = call "Get Next Event.vi"("Exit Event"="Exit", "event queue in"=w32) -> ("Condition (Exit:F)"=w34:bool, "next event"=w33:string, "event queue out"=w29:string[])  [unwired: 3 in]
    n6 = case shown="\"Load Last Config\"" w33 {
      tunnel: w31 -> [w37 w340 w377 w389 w395 w407 w434 w467 w493 w503 w519 w530 w538 w542 w550 w558 w564 w567 w583 w598 w604 w610 w615 w625 w668 w723 w753 w773 w785 w822 w832]
      tunnel: [w38 w339 w381 w388 w394 w406 w433 w466 w492 w503 w518 w529 w537 w541 w549 w557 w564 w567 w583 w597 w603 w610 w615 w626 w669 w722 w752 w773 w784 w822 w832] -> w30
      tunnel: [w42 w336 w378 w390 w398 w409 w436 w469 w498 w502 w509 w526 w534 w543 w551 w559 w566 w570 w591 w599 w605 w608 w621 w629 w661 w709 w736 w774 w783 w797 w833] -> w28
      tunnel: w29 -> [w41 w336 w378 w390 w398 w408 w435 w468 w498 w502 w508 w527 w533 w543 w551 w559 w565 w569 w592 w599 w605 w609 w621 w630 w662 w710 w735 w774 w782 w796 w833]
      tunnel: w26 -> [_ w331 _ _ _ _ _ _ _ _ _ _ _ _ _ _ _ _ _ _ _ _ _ _ _ _ _ _ _ _ _]
      tunnel: w25 -> [w36 _ _ _ _ _ _ _ _ _ _ _ _ _ _ _ _ _ _ _ _ _ w613 _ _ _ _ _ _ _ _]
      tunnel: w24 -> [w35 _ _ _ _ _ _ _ _ _ _ _ _ _ _ _ _ _ _ _ _ _ w611 _ _ _ _ _ _ _ _]
      frame "Main", Default {
        n7 = event shown="[0] Timeout" {
          selector: w36 -> [_ _ _ _ _ _ _ _ _ _ _ _ _ _ _ _ _ _ _ _ _ _ _ _ _ _ _]
          dyn-events: _ -> [_ _ _ _ _ _ _ _ _ _ _ _ _ _ _ _ _ _ _ _ _ _ _ _ _ _ _]
          timeout: 10 -> [_ _ _ _ _ _ _ _ _ _ _ _ _ _ _ _ _ _ _ _ _ _ _ _ _ _ _]
          tunnel: [w63 string[] ["Load"] string[] ["Load"] string[] ["Store Channel Group", "Save"] string[] ["Save"] string[] ["Store Channel Group", "Save As"] string[] ["Add Sensor"] string[] ["Delete Sensor"] string[] ["Store Channel Group", "Check for Sensor Select", "Check for Calibrate", "Check for Test Limits"] w118 string[] [] string[] [] string[] [] string[] ["Update DAQ Table"] string[] ["Update DAQ Table"] w252 string[] ["Update Fields"] string[] ["Update Fields"] string[] [] string[] [] string[] [] string[] [] string[] [] string[] [] string[] [] string[] [] string[] ["Part Config", "Update Channel Group"]] -> w40
          tunnel: w37 -> [w59 w92 w95 w97 w101 w104 w106 w108 w111 w123 w153 w163 w209 w223 w248 w254 w273 w278 w283 w288 w294 w300 w304 w309 w316 w320 w321]
          tunnel: [w64 w92 w94 w97 w100 w104 w106 w108 w110 w123 w153 w163 w208 w222 w247 w253 w272 w277 w282 w287 w293 w299 w303 w308 w315 w320 w321] -> w38
          tunnel: w37 -> [w67 _ _ _ _ _ _ _ _ _ _ _ _ _ _ w250 _ _ _ _ _ _ _ _ _ _ _]
          tunnel: w35 -> [_ _ _ _ _ _ _ _ _ _ _ _ _ _ _ _ _ _ _ _ _ _ _ _ _ _ _]
          event Timeout {
            n8 = event-data() -> ()  [unwired: 1 in, 1 out]
            n9 = Unbundle By Name(w67) -> ("Config Path"=w66:path, "Changes?"=w52:bool)
            "Config Path OUT" <- w66
            "Changes?" <- w52
            n10 = Unbundle By Name(w67) -> ("Calling VI Ref"=w60:refnum<vi>, "debug"=w68:bool)
            n11 = Empty String/Path?(string/path=w66) -> (empty?=w53:bool)
            n12 = Compound Arithmetic op=AND(w52, invert w53) -> (w65:bool)
            n13 = invoke class="VI" method="Ctrl Val.Get"(reference=w60, "Control Name"="DAQ Armed") -> (reference out=w45:refnum<vi>, "Get Control Value Variant"=w47:variant)  [unwired: 2 in, 2 out]
            n14 = invoke class="VI" method="Ctrl Val.Get"(reference=w45, "Control Name"="In O-scope Mode") -> ("Get Control Value Variant"=w50:variant)  [unwired: 2 in, 3 out]
            n15 = Variant To Data(type=FALSE, Variant=w47) -> (data=w44:bool)  [unwired: 1 in, 1 out]
            n16 = Variant To Data(type=FALSE, Variant=w50) -> (data=w43:bool)  [unwired: 1 in, 1 out]
            n17 = Or(x=w44, y=w43) -> (x .or. y?=w54:bool)
            n18 = case shown="False" w68 {
              tunnel: [w87 string[] []] -> w62
              tunnel: w60 -> [w86 _]
              frame False {
                n19 = property class="VI"(reference=w86) -> (error out=w84:errorcluster, "Exec.State"=w85:T20)  [unwired: 1 in, 1 out]
                n20 = call <vilib>:"Clear Errors.vi"("error in (no error)"=w84) -> ()  [unwired: 5 in, 2 out]
                n21 = case shown="\"Run top level\", \"Running\"" w85 {
                  tunnel: [string[] ["Exit"] string[] []] -> w87
                  frame Default {
                  }
                  frame "Run top level", "Running" {
                  }
                }
              }
              frame True {
              }
            }
            n22 = Select(t=2, s=w54, f=0) -> (s? t:f=w55:i32)
            n23 = property on="Open" class="Bool"("DisabledEnum"=w55) -> ()  [unwired: 2 in, 2 out]
            n24 = property on="Save As" class="Bool"("DisabledEnum"=w55) -> ()  [unwired: 2 in, 2 out]
            n25 = Bundle By Name(cluster=w59, "DAQ Running"=w54) -> (w58:T19)
            n26 = case shown="True" w65 {
              tunnel: [w69 w74] -> w64
              tunnel: w58 -> [w69 w73]
              tunnel: [string[] [] w72] -> w61
              tunnel: w54 -> [_ w71]
              frame False {
              }
              frame True {
                n27 = case shown="True" w71 {
                  tunnel: [w77 w82] -> w74
                  tunnel: w73 -> [w77 w83]
                  tunnel: [string[] [] string[] ["Load"]] -> w72
                  frame False {
                    w75 = T21."Enabled" ("Disabled")
                    n28 = property on="Save" class="Bool"("DisabledEnum"=w75) -> ()  [unwired: 2 in, 2 out]
                    n29 = property on="Revert" class="Bool"("DisabledEnum"=w75) -> ()  [unwired: 2 in, 2 out]
                    n30 = property on="Open" class="Bool"("DisabledEnum"=w75) -> ()  [unwired: 2 in, 2 out]
                    n31 = property on="Save As" class="Bool"("DisabledEnum"=w75) -> ()  [unwired: 2 in, 2 out]
                  }
                  frame True {
                    n32 = Bundle By Name(cluster=w83, "Changes?"=FALSE, "Revert"=TRUE) -> (w82:T19)
                    n33 = One Button Dialog(message="Can't make changes while DAQ is running.") -> ()  [unwired: 1 in, 1 out]
                  }
                }
              }
            }
            n34 = Build Array (concatenate)(w61, w62) -> (w63:string[])
          }
          event "Open": Value Change {
            n35 = event-data() -> ()  [unwired: 1 in, 1 out]
          }
          event "Revert": Value Change {
            n36 = event-data() -> ()  [unwired: 1 in, 1 out]
            n37 = Bundle By Name(cluster=w95, "Revert"="Revert") -> (w94:T19)
          }
          event "Save": Value Change {
            n38 = event-data() -> ()  [unwired: 1 in, 1 out]
          }
          event User Event {
            n39 = event-data() -> ("Graph Settings"=w99:T14)  [unwired: 1 in]
            n40 = Bundle By Name(cluster=w101, "Config.Graph Settings"=w99) -> (w100:T19)
          }
          event "Save As": Value Change {
            n41 = event-data() -> ()  [unwired: 1 in, 1 out]
          }
          event "Add Sensor": Value Change {
            n42 = event-data() -> ()  [unwired: 1 in, 1 out]
          }
          event "Delete Sensor": Value Change {
            n43 = event-data() -> ()  [unwired: 1 in, 1 out]
          }
          event Value Change {
            n44 = event-data() -> ()  [unwired: 1 in, 1 out]
            n45 = Bundle By Name(cluster=w111, "Channel Display"="Sensors", "Changes?"=TRUE) -> (w110:T19)
          }
          event "Header Table": Key Down? {
            n46 = event-data() -> ("CtlRef"=w116:refnum<vi>, "VKey"=w114:T22, "Char"=w115:i16)  [unwired: 1 in]
            n47 = case shown="\"Enter\", \"Return\", \"Down\"" w114 {
              tunnel: [1 ("Column") 1 ("Column") -1 ("Column")] -> w120
              tunnel: [FALSE TRUE TRUE] -> w119
              frame Default {
              }
              frame "Enter", "Return", "Down" {
              }
              frame "Up" {
              }
            }
            n48 = Equal?(x=w115, y=i16 9) -> (x = y?=w122:bool)
            n49 = Or(x=w119, y=w122) -> (x .or. y?=w117:bool)
            n50 = case shown="True" w117 {
              tunnel: w116 -> [_ w142]
              tunnel: w120 -> [_ w137]
              tunnel: [string[] [] string[] []] -> w118
              frame False {
              }
              frame True {
                n51 = property class="Tbl (strict)"(reference=w142) -> (reference out=w139:refnum<vi>, "EditPos"=w141:T23)  [unwired: 1 in, 1 out]
                n52 = Unbundle(w141) -> ("Row"=w136:i32)  [unwired: 1 out]
                n53 = Add(x=w137, y=w136) -> (x+y=w132:i32)
                n54 = In Range and Coerce(upper limit=3 ("y"), x=w132, lower limit=0) -> (coerced(x)=w135:i32)  [unwired: 1 out]
                n55 = Bundle("y"=w135, "Column"=0) -> (w140:cluster{"y":i32, "Column":i32})  [unwired: 1 in]
                n56 = property class="Tbl (strict)"(reference=w139, "EditPos"=w140) -> ()  [unwired: 1 in, 2 out]
              }
            }
            n57 = event-data("Discard?"=w117) -> ()  [unwired: 1 in, 1 out]
          }
          event "Header Table": Mouse Down {
            n58 = event-data() -> ("CtlRef"=w144:refnum<vi>)  [unwired: 1 in, 4 out]
            n59 = property class="Tbl (strict)"(reference=w144) -> (reference out=w143:refnum<vi>, "EditPos"=w145:T23)  [unwired: 1 in, 1 out]
            n60 = Unbundle(w145) -> ("Row"=w148:i32)  [unwired: 1 out]
            n61 = In Range and Coerce(upper limit=5 ("y"), x=w148, lower limit=0) -> (coerced(x)=w150:i32)  [unwired: 1 out]
            n62 = Bundle("y"=w150, "Column"=0) -> (w151:cluster{"y":i32, "Column":i32})  [unwired: 1 in]
            n63 = property class="Tbl (strict)"(reference=w143, "EditPos"=w151) -> ()  [unwired: 1 in, 2 out]
          }
          event "DAQ Table": Key Down? {
            n64 = event-data() -> ("CtlRef"=w156:refnum<vi>, "VKey"=w158:T22, "Char"=w159:i16)  [unwired: 1 in]
            n65 = case shown="\"Enter\", \"Return\", \"Down\"" w158 {
              tunnel: [1 ("Column") 1 ("Column") -1 ("Column")] -> w155
              tunnel: [FALSE TRUE TRUE] -> w160
              frame Default {
              }
              frame "Enter", "Return", "Down" {
              }
              frame "Up" {
              }
            }
            n66 = Equal?(x=w159, y=i16 9) -> (x = y?=w162:bool)
            n67 = Or(x=w160, y=w162) -> (x .or. y?=w157:bool)
            n68 = case shown="True" w157 {
              tunnel: w156 -> [_ w174]
              tunnel: w155 -> [_ w169]
              frame False {
              }
              frame True {
                n69 = property class="Tbl (strict)"(reference=w174) -> (reference out=w171:refnum<vi>, "EditPos"=w173:T23)  [unwired: 1 in, 1 out]
                n70 = Unbundle(w173) -> ("Row"=w168:i32)  [unwired: 1 out]
                n71 = case shown="2" w168 {
                  selector: w168 -> [_ w182 _ w191]
                  tunnel: w168 -> [w177 w180 _ _]
                  tunnel: w169 -> [w176 w179 w190 w196]
                  tunnel: [w175 w181 w185 w192] -> w167
                  frame Default {
                    n72 = Add(x=w176, y=w177) -> (x+y=w175:i32)
                  }
                  frame 2 {
                    n73 = Equal?(x=w179, y=-1) -> (x = y?=w183:bool)
                    n74 = Add(x=w180, y=w179) -> (x+y=w178:i32)
                    n75 = Select(t=w182, s=w183, f=w178) -> (s? t:f=w181:i32)
                  }
                  frame 5 {
                    n76 = Equal?(x=w190, y=-1) -> (x = y?=w189:bool)
                    n77 = Select(t=4, s=w189, f=7) -> (s? t:f=w185:i32)
                  }
                  frame 7 {
                    n78 = Equal?(x=w196, y=-1) -> (x = y?=w195:bool)
                    n79 = Select(t=5, s=w195, f=w191) -> (s? t:f=w192:i32)
                  }
                }
                n80 = In Range and Coerce(upper limit=7 ("y"), x=w167, lower limit=2) -> (coerced(x)=w166:i32)  [unwired: 1 out]
                n81 = Bundle("y"=w166, "Column"=0) -> (w172:cluster{"y":i32, "Column":i32})  [unwired: 1 in]
                n82 = property class="Tbl (strict)"(reference=w171, "EditPos"=w172) -> ()  [unwired: 1 in, 2 out]
              }
            }
            n83 = event-data("Discard?"=w157) -> ()  [unwired: 1 in, 1 out]
          }
          event "Header Table": Value Change {
            n84 = event-data() -> ()  [unwired: 1 in, 1 out]
            n85 = Index Array(array="Header Table", index (col)=0 ("disabled index (col)")) -> (element=w205:string[])  [unwired: 1 in]
            n86 = Array To Cluster(array=w205) -> (cluster=w203:T24)
            n87 = Bundle By Name(cluster=w209, "Config.Header"=w203, "Changes?"=TRUE) -> (w208:T19)
          }
          event "DAQ Table": Value Change {
            n88 = event-data() -> ()  [unwired: 1 in, 1 out]
            n89 = Index Array(array="DAQ Table", index (col)=0 ("disabled index (col)")) -> (element=w229:string[])  [unwired: 1 in]
            n90 = for {
              tunnel: w229 -> [w233] mode=indexing
              tunnel: [w231] -> w226 mode=indexing
              n91 = Match Pattern(string=w233, regular expression="[.]") -> (before substring=w239:string, after substring=w232:string, offset past match=w237:i32)  [unwired: 1 in, 1 out]
              n92 = Decimal Digit?(1:w239) -> (0:w238:bool)
              n93 = Equal?(x=w237, y=-1) -> (x = y?=w235:bool)
              n94 = Or(x=w238, y=w235) -> (x .or. y?=w234:bool)
              n95 = case shown="True" w234 {
                tunnel: [w241 w244] -> w231
                tunnel: w233 -> [_ w244]
                tunnel: w232 -> [w243 _]
                frame False {
                  n96 = Concatenate Strings("0." ("string"), w243) -> (w241:string)
                }
                frame True {
                }
              }
            }
            n97 = Index Array(array=w226, index #1=2 ("index"), index #5=7 ("index")) -> (element #1=w221:string, element #2=w219:string, element #3=w217:string, element #4=w215:string, element #5=w213:string)  [unwired: 3 in]
            n98 = Fract/Exp String To Number(string=w221) -> (number=w220:dbl)  [unwired: 3 in, 1 out]
            n99 = Decimal String To Number(string=w219) -> (number=w218:i32)  [unwired: 2 in, 1 out]
            n100 = Decimal String To Number(string=w217) -> (number=w216:i32)  [unwired: 2 in, 1 out]
            n101 = Fract/Exp String To Number(string=w215) -> (number=w214:dbl)  [unwired: 3 in, 1 out]
            n102 = Fract/Exp String To Number(string=w213) -> (number=w212:dbl)  [unwired: 3 in, 1 out]
            n103 = Bundle By Name(cluster=w223, "Config.DAQ Settings.Trigger Value"=w220, "Config.DAQ Settings.Trigger Samples"=w218, "Config.DAQ Settings.Pretrigger Samples"=w216, "Config.DAQ Settings.Trigger Interval"=w214, "Config.DAQ Settings.Sample Rate"=w212, "Changes?"=TRUE) -> (w222:T19)
          }
          event "Limit:": Value Change {
            n104 = event-data() -> ()  [unwired: 1 in, 1 out]
            n105 = Bundle By Name(cluster=w248, "Config.DAQ Settings.File Size Limit"="Limit:", "Changes?"=TRUE) -> (w247:T19)
          }
          event "DAQ Table": Mouse Down? {
            n106 = event-data() -> ("Coords"=w257:T25)  [unwired: 1 in]
            n107 = invoke on="DAQ Table" class="Tbl (strict)" method="Point To Row Column"("Point"=w257) -> ("CellPosition"=w256:T23)  [unwired: 5 in, 5 out]
            n108 = Unbundle By Name(w256) -> ("Row"=w255:i32)
            n109 = case shown="1" w255 {
              tunnel: w254 -> [w260 w266]
              tunnel: [w260 w265] -> w253
              tunnel: [string[] [] string[] ["Update DAQ Table"]] -> w252
              tunnel: [FALSE ("Discard?") TRUE ("Discard?")] -> w251
              tunnel: w250 -> [_ w261]
              frame 0, Default {
              }
              frame 1 {
                n110 = Unbundle By Name(w261) -> ("Config"=w267:T9)
                n111 = call "Select Analog Trigger Channel.vi"("Config"=w267) -> ("Config out"=w268:T9)  [unwired: 14 in]
                n112 = Bundle By Name(cluster=w266, "Config"=w268, "Changes?"=TRUE) -> (w265:T19)
              }
            }
            n113 = event-data("Discard?"=w251) -> ()  [unwired: 1 in, 1 out]
          }
          event "Trigger Type": Value Change {
            n114 = event-data() -> ()  [unwired: 1 in, 1 out]
            n115 = Bundle By Name(cluster=w273, "Config.DAQ Settings.Trigger Type"="Trigger Type", "Changes?"=TRUE) -> (w272:T19)
          }
          event "Save Mode": Value Change {
            n116 = event-data() -> ()  [unwired: 1 in, 1 out]
            n117 = Bundle By Name(cluster=w278, "Config.DAQ Settings.Save Mode"="Save Mode", "Changes?"=TRUE) -> (w277:T19)
          }
          event "Trigger Stop Method": Value Change {
            n118 = event-data() -> ()  [unwired: 1 in, 1 out]
            n119 = Bundle By Name(cluster=w283, "Config.DAQ Settings.Trigger Stop Method"="Trigger Stop Method", "Changes?"=TRUE) -> (w282:T19)
          }
          event Value Change {
            n120 = event-data() -> ()  [unwired: 1 in, 1 out]
            n121 = Bundle By Name(cluster=w288, "Config.DAQ Settings.Log File Type"="Log File Type", "Changes?"=TRUE) -> (w287:T19)
          }
          event "Minutes": Value Change {
            n122 = event-data() -> ()  [unwired: 1 in, 1 out]
            n123 = Not(x="Minutes") -> (.not. x?=w290:bool)
            n124 = Bundle By Name(cluster=w294, "Changes?"=TRUE, "Config.DAQ Settings.Time Units"=w290) -> (w293:T19)
            n125 = local write "Hours"(w290) -> ()
          }
          event "Hours": Value Change {
            n126 = event-data() -> ()  [unwired: 1 in, 1 out]
            n127 = Not(x="Hours") -> (.not. x?=w297:bool)
            n128 = Bundle By Name(cluster=w300, "Changes?"=TRUE, "Config.DAQ Settings.Time Units"="Hours") -> (w299:T19)
            n129 = local write "Minutes"(w297) -> ()
          }
          event "Sample Sec": Value Change {
            # "False = Sec\nTrue = Min"
            n130 = event-data() -> ()  [unwired: 1 in, 1 out]
            n131 = Not(x="Sample Sec") -> (.not. x?=w301:bool)
            n132 = local write "Sample Min"(w301) -> ()
            n133 = Bundle By Name(cluster=w304, "Changes?"=TRUE, "Config.DAQ Settings.Rate Sec/Min"=w301) -> (w303:T19)
          }
          event "Sample Min": Value Change {
            # "False = Sec\nTrue = Min"
            n134 = event-data() -> ()  [unwired: 1 in, 1 out]
            n135 = Not(x="Sample Min") -> (.not. x?=w311:bool)
            n136 = local write "Sample Sec"(w311) -> ()
            n137 = Bundle By Name(cluster=w309, "Changes?"=TRUE, "Config.DAQ Settings.Rate Sec/Min"="Sample Min") -> (w308:T19)
          }
          event "Auto Save": Value Change {
            n138 = event-data() -> ()  [unwired: 1 in, 1 out]
            n139 = Bundle By Name(cluster=w316, "Config.DAQ Settings.Auto Save"="Auto Save", "Changes?"=TRUE) -> (w315:T19)
          }
          event Mouse Leave {
            w318 = FALSE ("Key Focus")
            n140 = event-data() -> ()  [unwired: 1 in, 4 out]
            n141 = property on="Header Table" class="Tbl (strict)"("Key Focus"=w318) -> ()  [unwired: 2 in, 2 out]
            n142 = property on="DAQ Table" class="Tbl (strict)"("Key Focus"=w318) -> ()  [unwired: 2 in, 2 out]
            n143 = property on="Description" class="Str"("Key Focus"=w318) -> ()  [unwired: 2 in, 2 out]
          }
          event "Part Config": Value Change {
            n144 = event-data() -> ()  [unwired: 1 in, 1 out]
            n145 = property on="Part Config" class="Bool (strict)"("Value"=FALSE ("Part Config Wizard")) -> ()  [unwired: 2 in, 2 out]
          }
        }
        n146 = call "Insert Multiple Events.vi"("Events to Insert"=w40, "Event queue in"=w41) -> ("Event queue out"=w42:string[])  [unwired: 5 in]
      }
      frame "Init" {
        # "On initialization, load the list of available channels from the system.ini file."
        n147 = Unbundle By Name(w340) -> ("App Path"=w324:path, "Config"=w334:T9)
        n148 = Not Equal?(x=w331, y=path "") -> (x != y?=w328:bool)
        n149 = case shown="False" w328 {
          tunnel: w331 -> [_ w371]
          tunnel: w334 -> [w350 w372]
          tunnel: [w349 w370] -> w333
          tunnel: w324 -> [_ _]
          tunnel: [path "" ("Sensor Config Path") w371] -> w332
          frame False {
            n150 = for {
              tunnel: T12 {"Channel"="", "Type"="", "Acquire"=FALSE, "Name"="", "Sensor"="", "Data Index"=0} ("Channel") -> [w357]
              tunnel: string[] ["9221_AI-00", "9221_AI-01", "9221_AI-02", "9221_AI-03", "9221_AI-04", "9221_AI-05", "9221_AI-06", "9221_AI-07", "9205_AI-00", "9205_AI-01", "9205_AI-02", "9205_AI-03", "9205_AI-04", "9205_AI-05", "9205_AI-06", "9205_AI-07", "9208_AI-00", "9208_AI-01", "9208_AI-02", "9208_AI-03", "9208_AI-04", "9208_AI-05", "9208_AI-06", "9208_AI-07", "9211_TC-00", "9211_TC-01", "9211_TC-02", "9211_TC-03"] ("Strings []") -> [w354] mode=indexing
              tunnel: [w356] -> w347 mode=indexing
              tunnel: [T15 {"Channel Acquired?"=FALSE, "RMS?"=FALSE, "Pk-Pk"=FALSE, "Frequency"=FALSE, "EU High Limit 1"=0.0, "EU Low Limit 1"=0.0, "EU High Limit 2"=0.0, "EU Low Limit 2"=0.0, "RMS High Limit"=0.0, "RMS Low Limit"=0.0, "Pk-Pk High Limit "=0.0, "Pk-Pk Low Limit"=0.0, "Frequency High Limit"=0.0, "Frequency Low Limit"=0.0} ("Test Limit")] -> w344 mode=indexing
              i -> [w351]
              n151 = case shown="24..27" w351 {
                tunnel: ["Direct Connection" ("Sensor") "Direct Connection" ("Sensor") "Direct Connection" ("Sensor") "Direct T-Type Thermocouple" ("Sensor")] -> w353
                tunnel: ["0-60 VDC" ("Sensor") "0-10 VDC" ("Sensor") "0-20 mA" ("Sensor") "T-Type" ("Sensor")] -> w352
                frame 0..7, Default {
                }
                frame 8..15 {
                }
                frame 16..23 {
                }
                frame 24..27 {
                }
              }
              n152 = Bundle By Name(cluster=w357, "Channel"=w354, "Type"=w352, "Sensor"=w353, "Data Index"=w351) -> (w356:T12)
            }
            n153 = local write "Config Name"("Sample" ("Config Name")) -> ()
            n154 = Bundle By Name(cluster=w350, "Channels"=w347, "DAQ Settings.Auto Save"=TRUE, "Test Limits"=w344, "DAQ Settings.Log File Type"=Log_File_Type."Basic") -> (w349:T9)
          }
          frame True {
            n155 = call "Read Characters From File with Error Out.vi"("file path (dialog if empty)"=w371) -> ("character string"=w373:string)  [unwired: 10 in, 4 out]
            n156 = Unflatten From String(type=w372, binary string=w373) -> (value=w370:T9)  [unwired: 3 in, 2 out]
            n157 = Unbundle By Name(w370) -> ("Header"=w369:T13)
            n158 = Cluster To Array(cluster=w369) -> (array=w368:string[])
            n159 = Build Array(w368) -> (w367:string[][])
            n160 = Transpose 2D Array(2D array=w367) -> (transposed array=w366:string[][])
            n161 = local write "Header Table"(w366) -> ()
          }
        }
        n162 = Build Path(base path=w324, name or relative path="Configurations") -> (appended path=w329:path)
        n163 = Build Path(base path=w324, name or relative path="App Config.ini") -> (appended path=w325:path)
        n164 = Bundle By Name(cluster=w340, "config start path"=w329, "Config Path"=w331, "Config"=w333, "Config Saved"=w333, "debug"=FALSE, "App Config Path"=w325) -> (w339:T19)
        n165 = Current VI's Path() -> (path=w338:path)
        n166 = call "Set Window Title using Path.vi"("VI path"=w338, "File Path"=w332, "Title"="Sensor Configuration") -> ()  [unwired: 12 in, 1 out]
      }
      frame "Load Sensors" {
        n167 = Unbundle By Name(w377) -> ("Cal Base Path"=w376:path)
        n168 = Build Path(base path=w376, name or relative path="Sensors.scl") -> (appended path=w380:path)
        n169 = call "Open Sensor Library.vi"("Sensor Library Path"=w380) -> ("Sensors Info"=w375:T18)  [unwired: 4 in, 2 out]
        n170 = disable-structure shown="Enabled" {
          disable-tunnel: w375 -> [w383 w384]
          disable-tunnel: [w382 w384] -> w374
          frame Disabled {
            n171 = call "Add Current Sensors.vi"("Sensors Info IN"=w383) -> ("Sensors Info OUT"=w382:T18)  [unwired: 10 in]
          }
          frame Enabled {
          }
        }
        n172 = Bundle By Name(cluster=w377, "Sensors"=w374) -> (w381:T19)
      }
      frame "Store Channel Group" {
        n173 = Unbundle By Name(w389) -> ("Config"=w387:T9, "Channel Display"=w386:T7)
        n174 = call "Store Channel Display.vi"("Channels in"=w387, "Channel Display"=w386) -> ("Channels out"=w385:T9)  [unwired: 13 in]
        n175 = Bundle By Name(cluster=w389, "Config"=w385) -> (w388:T19)
      }
      frame "Update Channel Group" {
        n176 = Unbundle By Name(w395) -> ("Sensors"=w397:T18, "Config.Channels"=w396:T12[], "Config.Graph Settings"=w391:T14)
        n177 = call "Update Channel Display.vi"("Sensors"=w397, "Channels"=w396, "Config.Graph Settings"=w391) -> ("Graph Settings"=w392:T14, "Sensors 2"=w393:T7)  [unwired: 11 in]
        n178 = local write "Sensors"(w393) -> ()
        n179 = Bundle By Name(cluster=w395, "Channel Display"=w393, "Config.Graph Settings"=w392) -> (w394:T19)
      }
      frame "Check for Sensor Select" {
        n180 = Unbundle By Name(w407) -> ("Channel Display"=w402:T7)
        n181 = for {
          tunnel: w402 -> [w424] mode=indexing
          tunnel: [w423] -> w400 mode=indexing
          n182 = Unbundle By Name(w424) -> ("Chg Sensor"=w423:bool)
        }
        n183 = Or Array Elements(Boolean array=w400) -> (logical OR=w403:bool)
        n184 = Search 1D Array(1D array=w400, element=TRUE) -> (index of element=w399:i32)  [unwired: 1 in]
        n185 = case shown="True" w403 {
          tunnel: w400 -> [_ w415]
          tunnel: [-1 ("index of element") w414] -> w405
          tunnel: [string[] [] ("Events to Insert") w413] -> w404
          tunnel: w399 -> [_ w412]
          frame False {
          }
          frame True {
            n186 = case shown="24..27" w412 {
              tunnel: w415 -> [w419 _]
              tunnel: [w418 -1 ("index of element")] -> w414
              tunnel: [string[] ["Change Sensor", "Clear Change Sensor Buttons", "Store Channel Group", "Update Channel Group"] ("Events to Insert") string[] ["Clear Change Sensor Buttons"] ("Events to Insert")] -> w413
              frame Default {
                n187 = Search 1D Array(1D array=w419, element=TRUE) -> (index of element=w418:i32)  [unwired: 1 in]
              }
              frame 24..27 {
                n188 = One Button Dialog(message="Thermocouple Channels cannot\nhave sensors assigned to them.") -> ()  [unwired: 1 in, 1 out]
              }
            }
          }
        }
        n189 = Bundle By Name(cluster=w407, "Channel Select"=w405) -> (w406:T19)
        n190 = call "Insert Multiple Events.vi"("Events to Insert"=w404, "Event queue in"=w408) -> ("Event queue out"=w409:string[])  [unwired: 5 in]
      }
      frame "Check for Calibrate" {
        n191 = Unbundle By Name(w434) -> ("Channel Display"=w429:T7)
        n192 = for {
          tunnel: w429 -> [w458] mode=indexing
          tunnel: [w457] -> w426 mode=indexing
          tunnel: [w456] -> w425 mode=indexing
          n193 = Unbundle By Name(w458) -> ("Cal"=w457:bool, "Sensor"=w456:string)
        }
        n194 = Or Array Elements(Boolean array=w426) -> (logical OR=w430:bool)
        n195 = Search 1D Array(1D array=w426, element=TRUE) -> (index of element=w427:i32)  [unwired: 1 in]
        n196 = case shown="True" w430 {
          tunnel: [-1 ("index of element") w442] -> w432
          tunnel: [string[] [] ("Events to Insert") w441] -> w431
          tunnel: w427 -> [_ w440]
          tunnel: w425 -> [_ w439]
          frame False {
          }
          frame True {
            n197 = case shown="Default" w440 {
              selector: w440 -> [w444 _]
              tunnel: [w446 -1 ("index of element")] -> w442
              tunnel: [w447 string[] ["Clear Calibrate Buttons"] ("Events to Insert")] -> w441
              tunnel: w439 -> [w445 _]
              frame Default {
                n198 = Index Array(array=w445, index=w444) -> (element=w443:string)
                n199 = case shown="\"Direct Connection\"" w443 {
                  tunnel: [string[] ["Store Channel Group", "Calibrate Sensor", "Clear Calibrate Buttons", "Update Channel Group"] ("Events to Insert") string[] ["Clear Calibrate Buttons"] ("Events to Insert")] -> w447
                  tunnel: [w448 -1 ("index of element")] -> w446
                  tunnel: w444 -> [w448 _]
                  frame Default {
                  }
                  frame "Direct Connection" {
                    n200 = One Button Dialog(message="This sensor type is fixed and\ncannot be calibrated.") -> ()  [unwired: 1 in, 1 out]
                  }
                }
              }
              frame 24..27 {
                n201 = One Button Dialog(message="Thermocouple Channels cannot\nbe calibrated.") -> ()  [unwired: 1 in, 1 out]
              }
            }
          }
        }
        n202 = Bundle By Name(cluster=w434, "Channel Select"=w432) -> (w433:T19)
        n203 = call "Insert Multiple Events.vi"("Events to Insert"=w431, "Event queue in"=w435) -> ("Event queue out"=w436:string[])  [unwired: 5 in]
      }
      frame "Check for Test Limits" {
        # "Determine Which Test Limits button is selected"
        n204 = Unbundle By Name(w467) -> ("Channel Display"=w462:T7)
        n205 = for {
          tunnel: w462 -> [w484] mode=indexing
          tunnel: [w483] -> w460 mode=indexing
          n206 = Unbundle By Name(w484) -> ("Test Limits"=w483:bool)
        }
        n207 = Or Array Elements(Boolean array=w460) -> (logical OR=w463:bool)
        n208 = Search 1D Array(1D array=w460, element=TRUE) -> (index of element=w459:i32)  [unwired: 1 in]
        n209 = case shown="True" w463 {
          tunnel: w460 -> [_ w475]
          tunnel: [-1 ("index of element") w474] -> w465
          tunnel: [string[] [] ("Events to Insert") w473] -> w464
          tunnel: w459 -> [_ w472]
          frame False {
          }
          frame True {
            n210 = case shown="Default" w472 {
              tunnel: w475 -> [w479 _]
              tunnel: [w478 -1 ("index of element")] -> w474
              tunnel: [string[] ["Store Channel Group", "Test Limits", "Clear Test Limits Buttons", "Update Channel Group"] ("Events to Insert") string[] ["Clear Calibrate Buttons"] ("Events to Insert")] -> w473
              frame Default {
                n211 = Search 1D Array(1D array=w479, element=TRUE) -> (index of element=w478:i32)  [unwired: 1 in]
              }
              frame 24..27 {
                n212 = One Button Dialog(message="Thermocouple Channels cannot\nbe calibrated.") -> ()  [unwired: 1 in, 1 out]
              }
            }
          }
        }
        n213 = Bundle By Name(cluster=w467, "Channel Select"=w465) -> (w466:T19)
        n214 = call "Insert Multiple Events.vi"("Events to Insert"=w464, "Event queue in"=w468) -> ("Event queue out"=w469:string[])  [unwired: 5 in]
      }
      frame "Change Sensor" {
        n215 = Unbundle By Name(w493) -> ("Channel Display"=w496:T7, "Channel Select"=w497:i32, "Sensors"=w485:T18)
        n216 = Index Array(array=w496, index=w497) -> (element=w495:T8)
        n217 = Unbundle By Name(w495) -> ("Channel"=w489:string, "Sensor"=w487:string)
        n218 = call "Select Sensor.vi"("Channel"=w489, "Sensor Name in"=w487, "Sensors"=w485) -> ("Sensor Name out"=w488:string)  [unwired: 12 in]
        n219 = Bundle By Name(cluster=w495, "Sensor"=w488) -> (w494:T8)
        n220 = Replace Array Subset(array=w496, new element=w494, index=w497) -> (w491:T7)
        n221 = for {
          tunnel: w491 -> [w501] mode=indexing
          tunnel: [w500] -> w490 mode=indexing
          tunnel: FALSE ("Chg Sensor") -> [w499]
          n222 = Bundle By Name(cluster=w501, "Chg Sensor"=w499) -> (w500:T8)
        }
        n223 = local write "Sensors"(w490) -> ()
        n224 = Bundle By Name(cluster=w493, "Channel Display"=w490) -> (w492:T19)
      }
      frame "Change Analog Trigger" {
      }
      frame "Calibrate Sensor" {
        n225 = Unbundle By Name(w519) -> ("TCP Stream Ref"=w504:refnum<vi>, "Sensors"=w516:T18, "Channel Display"=w522:T7, "Channel Select"=w512:i32, "Cal Base Path"=w511:path, "System"=w505:T1)
        n226 = for {
          tunnel: w516 -> [w524] mode=indexing
          tunnel: [w523] -> w515 mode=indexing
          n227 = Unbundle By Name(w524) -> ("Sensor Name"=w523:string)
        }
        n228 = Index Array(array=w522, index=w512) -> (element=w521:T8)
        n229 = Unbundle By Name(w521) -> ("Sensor"=w514:string)
        n230 = Search 1D Array(1D array=w515, element=w514) -> (index of element=w513:i32)  [unwired: 1 in]
        n231 = Index Array(array=w516, index=w513) -> (element=w520:T26)
        n232 = call "Calibrate Sensor.vi"("Sensor"=w520, "System"=w505, "TCP Stream Ref"=w504, "Channel Info"=w521, "Cal Base Path"=w511, "Channel index"=w512) -> ("Sensor out"=w506:T26, "OK Out"=w507:bool)  [unwired: 8 in]
        n233 = Replace Array Subset(array=w516, new element=w506, index=w513) -> (w517:T18)
        n234 = call "Insert Multiple Events.vi"("Insert all? (T)"=w507, "Events to Insert"=string[] ["Save scaling sensors"], "Event queue in"=w508) -> ("Event queue out"=w509:string[])  [unwired: 4 in]
        n235 = Bundle By Name(cluster=w519, "Sensors"=w517) -> (w518:T19)
      }
      frame "Add Sensor" {
        n236 = Unbundle By Name(w530) -> ("Sensors"=w531:T18)
        n237 = call "Add Sensor.vi"("Sensors in"=w531) -> ("Sensors out"=w528:T18)  [unwired: 13 in, 1 out]
        n238 = call "Insert Multiple Events.vi"("Events to Insert"=string[] ["Save scaling sensors"], "Event queue in"=w527) -> ("Event queue out"=w526:string[])  [unwired: 5 in]
        n239 = Bundle By Name(cluster=w530, "Sensors"=w528) -> (w529:T19)
      }
      frame "Delete Sensor" {
        # "delete sensor from list"
        n240 = Unbundle By Name(w538) -> ("Sensors"=w536:T18)
        n241 = call "Delete Sensor.vi"("Sensors"=w536) -> ("Sensors out"=w535:T18)  [unwired: 14 in]
        n242 = Bundle By Name(cluster=w538, "Sensors"=w535) -> (w537:T19)
        n243 = call "Insert Multiple Events.vi"("Events to Insert"=string[] ["Save scaling sensors", "Update Channel Group"], "Event queue in"=w533) -> ("Event queue out"=w534:string[])  [unwired: 5 in]
      }
      frame "Clear Change Sensor Buttons" {
        n244 = Unbundle By Name(w542) -> ("Channel Display"=w539:T7)
        n245 = for {
          tunnel: w539 -> [w546] mode=indexing
          tunnel: [w545] -> w540 mode=indexing
          n246 = Bundle By Name(cluster=w546, "Chg Sensor"=FALSE) -> (w545:T8)
        }
        n247 = Bundle By Name(cluster=w542, "Channel Display"=w540) -> (w541:T19)
        n248 = local write "Sensors"(w540) -> ()
      }
      frame "Clear Calibrate Buttons" {
        n249 = Unbundle By Name(w550) -> ("Channel Display"=w548:T7)
        n250 = for {
          tunnel: w548 -> [w554] mode=indexing
          tunnel: [w553] -> w547 mode=indexing
          n251 = Bundle By Name(cluster=w554, "Cal"=FALSE ("Chg Sensor")) -> (w553:T8)
        }
        n252 = local write "Sensors"(w547) -> ()
        n253 = Bundle By Name(cluster=w550, "Channel Display"=w547) -> (w549:T19)
      }
      frame "Clear Test Limits Buttons" {
        n254 = Unbundle By Name(w558) -> ("Channel Display"=w556:T7)
        n255 = for {
          tunnel: w556 -> [w562] mode=indexing
          tunnel: [w561] -> w555 mode=indexing
          n256 = Bundle By Name(cluster=w562, "Test Limits"=FALSE ("Chg Sensor")) -> (w561:T8)
        }
        n257 = local write "Sensors"(w555) -> ()
        n258 = Bundle By Name(cluster=w558, "Channel Display"=w555) -> (w557:T19)
      }
      frame "Close" {
        n259 = call "Insert Multiple Events.vi"("Events to Insert"=string[] ["Store Channel Group", "Check For Changes"], "Event queue in"=w565) -> ("Event queue out"=w566:string[])  [unwired: 5 in]
      }
      frame "Check For Changes" {
        n260 = Unbundle By Name(w567) -> ("Config"=w573:T9, "Config Saved"=w572:T9)
        n261 = Not Equal?(x=w573, y=w572) -> (x != y?=w571:bool)
        n262 = case shown="False" w571 {
          tunnel: [string[] ["Exit"] ("Events to Insert") w577] -> w568
          frame False {
          }
          frame True {
            n263 = Two Button Dialog(message="Sensor Configuration has changed.\nDo you want to save changes?", 1:"No" ("F button name (\"Cancel\")"), 2:"Yes" ("T button name (\"OK\")")) -> (T button?=w580:bool)
            n264 = Select(t=string[] ["Save", "Exit"] ("Events to Insert"), s=w580, f=string[] ["Exit"] ("Events to Insert")) -> (s? t:f=w577:string[])
          }
        }
        n265 = call "Insert Multiple Events.vi"("Events to Insert"=w568, "Event queue in"=w569) -> ("Event queue out"=w570:string[])  [unwired: 5 in]
      }
      frame "Save scaling sensors" {
        # "insert into queue"
        # "save scaling sensor values"
        n266 = Unbundle By Name(w583) -> ("Cal Base Path"=w582:path, "Sensors"=w586:T18)
        n267 = Build Path(base path=w582, name or relative path="Sensors.scl") -> (appended path=w587:path)
        n268 = Flatten To String(anything=w586) -> (data string=w585:string)  [unwired: 3 in, 2 out]
        n269 = call "Write Characters To File with Advisory Dialog Option and Error Out.vi"("file path (dialog if empty)"=w587, "character string"=w585, "advisory dialog? (display:T)"=FALSE) -> ()  [unwired: 11 in, 2 out]
        n270 = call "Insert Multiple Events.vi"("Insert all? (T)"=FALSE, "Events to Insert"=string[] [], "Event queue in"=w592) -> ("Event queue out"=w591:string[])  [unwired: 4 in]
      }
      frame "Test Limits" {
        n271 = Unbundle By Name(w598) -> ("Config"=w596:T9, "Channel Select"=w595:i32, "Sensors"=w594:T18)
        n272 = call "Test Limits.vi"("Config In"=w596, "Channel Select"=w595, "Sensors"=w594) -> ("Config Out"=w593:T9)  [unwired: 12 in]
        n273 = Bundle By Name(cluster=w598, "Config"=w593) -> (w597:T19)
      }
      frame "Part Config" {
        n274 = Unbundle By Name(w604) -> ("Config"=w602:T9)
        n275 = call "Part Config.vi"("Loaded Config"=w602) -> ("Config Out"=w601:T9, "Changes?"=w600:bool)  [unwired: 13 in]
        n276 = Bundle By Name(cluster=w604, "Config"=w601, "Changes?"=w600) -> (w603:T19)
      }
      frame "Blank" {
        # "insert into queue"
        # "blank case template"
        n277 = call "Insert Multiple Events.vi"("Insert all? (T)"=TRUE, "Events to Insert"=string[] [], "Event queue in"=w609) -> ("Event queue out"=w608:string[])  [unwired: 4 in]
      }
      frame "Exit" {
        n278 = Unregister For Events(event registration refnum=w613) -> (error out=w612:errorcluster)  [unwired: 1 in]
        n279 = Destroy User Event(user event=w611, error in=w612) -> ()  [unwired: 1 out]
        n280 = Unbundle By Name(w615) -> ("Cal Base Path"=w614:path, "Sensors"=w618:T18)
        n281 = Flatten To String(anything=w618) -> (data string=w617:string)  [unwired: 3 in, 2 out]
        n282 = Build Path(base path=w614, name or relative path="Sensors.scl") -> (appended path=w619:path)
        n283 = call "Write Characters To File with Advisory Dialog Option and Error Out.vi"("file path (dialog if empty)"=w619, "character string"=w617, "advisory dialog? (display:T)"=FALSE) -> ()  [unwired: 11 in, 2 out]
      }
      frame "Load Last Config" {
        n284 = Unbundle By Name(w625) -> ("App Path"=w623:path, "App Config Path"=w624:path)
        n285 = call "Read App Config.vi"("App Config Path"=w624) -> ("Last Config"=w622:path)  [unwired: 13 in, 5 out]
        n286 = Empty String/Path?(string/path=w622) -> (empty?=w627:bool)
        n287 = case shown="True" w627 {
          tunnel: [string[] ["Load"] w642] -> w628
          tunnel: w625 -> [w633 w638]
          tunnel: [w632 w637] -> w626
          tunnel: w622 -> [w631 _]
          tunnel: w623 -> [_ w641]
          frame False {
            # "There is a last config in the the ini file."
            n288 = Bundle By Name(cluster=w633, "Config Path"=w631) -> (w632:T19)
          }
          frame True {
            # "NO config defined in INI file, so check if the sample config is available."
            n289 = Build Path(base path=w641, name or relative path="Configurations\\Sample.cfg") -> (appended path=w639:path)
            n290 = call <vilib>:"Check if File or Folder Exists.vi"("path"=w639) -> ("file or folder exists?"=w636:bool, "dup path"=w635:path)  [unwired: 8 in, 1 out]
            n291 = case shown="True" w636 {
              tunnel: [string[] [] string[] ["Load", "Remember Config"]] -> w642
              tunnel: w638 -> [w644 w647]
              tunnel: [w644 w646] -> w637
              tunnel: w635 -> [_ w645]
              frame False {
                # "The sample config is NOT available."
              }
              frame True {
                # "The sample config is available."
                n292 = Bundle By Name(cluster=w647, "Config Path"=w645) -> (w646:T19)
              }
            }
          }
        }
        n293 = call "Insert Multiple Events.vi"("Events to Insert"=w628, "Event queue in"=w630) -> ("Event queue out"=w629:string[])  [unwired: 5 in]
      }
      frame "Load" {
        n294 = Unbundle By Name(w668) -> ("Calling VI Ref"=w658:refnum<vi>, "Revert"=w659:bool, "Config Path"=w652:path, "config start path"=w656:path, "Config"=w665:T9, "Load Prompt"=w649:bool)
        n295 = Empty String/Path?(string/path=w652) -> (empty?=w654:bool)
        n296 = Not A Number/Path/Refnum?(number/path/refnum=w652) -> (NaN/Path/Refnum?=w653:bool)
        n297 = Or(x=w654, y=w653) -> (x .or. y?=w651:bool)
        n298 = Select(t=w656, s=w651, f=w652) -> (s? t:f=w655:path)
        n299 = case shown="False" w659 {
          tunnel: [w674 w682] -> w667
          tunnel: [w673 w681] -> w666
          tunnel: [w672 w680] -> w664
          tunnel: "*.cfg" ("[pattern]") -> [w671 w679]
          tunnel: w655 -> [_ w677]
          tunnel: w652 -> [w670 _]
          tunnel: w649 -> [_ w678]
          frame True {
            n300 = call "Read Characters From File with Error Out.vi"("file path (dialog if empty)"=w670, "[pattern]"=w671) -> ("new file path (NotAPath if cancelled)"=w673:path, "character string"=w672:string, "error out"=w674:errorcluster)  [unwired: 9 in, 2 out]
          }
          frame False {
            n301 = Select(t=path "", s=w678, f=w677) -> (s? t:f=w676:path)
            n302 = call "Read Characters From File with Error Out.vi"("file path (dialog if empty)"=w676, "start path (Not A Path)"=w677, "[pattern]"=w679) -> ("new file path (NotAPath if cancelled)"=w681:path, "character string"=w680:string, "error out"=w682:errorcluster)  [unwired: 8 in, 2 out]
          }
        }
        n303 = property class="VI"(reference=w658) -> ("Path"=w657:path)  [unwired: 1 in, 2 out]
        n304 = case shown="No Error" w667 {
          tunnel: w668 -> [w702 w705]
          tunnel: [w701 w704] -> w669
          tunnel: w666 -> [w690 _]
          tunnel: w665 -> [w700 _]
          tunnel: w664 -> [w699 _]
          tunnel: [w696 _] -> _
          tunnel: w657 -> [w687 _]
          tunnel: [string[] ["Update Channel Group", "Update DAQ Table", "Remember Config"] ("event queue out") string[] [] ("event queue out")] -> w650
          frame No Error {
            w685 = T21."Disabled and Grayed Out" ("Disabled")
            w686 = FALSE ("Revert")
            n305 = Unflatten From String(type=w700, binary string=w699) -> (value=w697:T9, error out=w695:errorcluster)  [unwired: 3 in, 1 out]
            n306 = Unbundle(w695) -> ("status"=w696:bool)  [unwired: 2 out]
            n307 = Unbundle By Name(w697) -> ("Header"=w691:T13)
            n308 = local write "Changes Latch"(TRUE ("Changes Latch")) -> ()
            n309 = Strip Path(path=w690) -> (name=→"Config Name":string)  [unwired: 1 out]
            n310 = Cluster To Array(cluster=w691) -> (array=w694:string[])
            n311 = property on="Revert" class="Bool"("DisabledEnum"=w685) -> ()  [unwired: 2 in, 2 out]
            n312 = property on="Save" class="Bool"("DisabledEnum"=w685) -> ()  [unwired: 2 in, 2 out]
            n313 = call "Set Window Title using Path.vi"("VI path"=w687, "File Path"=w690, "Title"="Configuration") -> ()  [unwired: 12 in, 1 out]
            n314 = Build Array(w694) -> (w693:string[][])
            n315 = Bundle By Name(cluster=w702, "Load Prompt"=TRUE, "Config Path"=w690, "Config"=w697, "Revert"=w686, "Changes?"=w686) -> (w701:T19)
            n316 = Transpose 2D Array(2D array=w693) -> (transposed array=w692:string[][])
            n317 = local write "Header Table"(w692) -> ()
          }
          frame Error {
            n318 = Bundle By Name(cluster=w705, "Load Prompt"=TRUE) -> (w704:T19)
          }
        }
        n319 = call "Insert Multiple Events.vi"("Insert all? (T)"=TRUE ("Insert?"), "Events to Insert"=w650, "Event queue in"=w662) -> ("Event queue out"=w661:string[])  [unwired: 4 in]
      }
      frame "Save As" {
        n320 = Unbundle By Name(w723) -> ("Config Saved"=w713:T9, "Config Path"=w707:path, "Config"=w721:T9, "Channel Display"=w720:T7, "Changes?"=w711:bool)
        n321 = call "Store Channel Display.vi"("Channels in"=w721, "Channel Display"=w720) -> ("Channels out"=w714:T9)  [unwired: 13 in]
        n322 = Flatten To String(anything=w714) -> (data string=w726:string)  [unwired: 3 in, 2 out]
        n323 = call "Write Characters To File with Advisory Dialog Option and Error Out.vi"("character string"=w726, "pattern"="*.cfg") -> ("new file path (Not A Path if cancelled)"=w724:path, "error out"=w725:errorcluster)  [unwired: 12 in]
        n324 = case shown="No Error" w725 {
          tunnel: w724 -> [w729 _]
          tunnel: [w729 w734] -> w719
          tunnel: w707 -> [_ w734]
          tunnel: [w731 w733] -> w715
          tunnel: w714 -> [w731 _]
          tunnel: w713 -> [_ w733]
          tunnel: [FALSE w732] -> w712
          tunnel: w711 -> [_ w732]
          frame No Error {
            w727 = T21."Disabled and Grayed Out" ("Disabled")
            n325 = Strip Path(path=w729) -> (name=w728:string)  [unwired: 1 out]
            n326 = local write "Config Name"(w728) -> ()
            n327 = property on="Save" class="Bool"("DisabledEnum"=w727) -> ()  [unwired: 2 in, 2 out]
            n328 = property on="Revert" class="Bool"("DisabledEnum"=w727) -> ()  [unwired: 2 in, 2 out]
          }
          frame Error {
          }
        }
        n329 = Current VI's Path() -> (path=w718:path)
        n330 = Bundle By Name(cluster=w723, "Config Saved"=w715, "Config Path"=w719, "Changes?"=w712) -> (w722:T19)
        n331 = call "Insert Multiple Events.vi"("Events to Insert"=string[] ["Remember Config"], "Event queue in"=w710) -> ("Event queue out"=w709:string[])  [unwired: 5 in]
        n332 = call "Set Window Title using Path.vi"("VI path"=w718, "File Path"=w719, "Title"="Sensor Configuration") -> ()  [unwired: 12 in, 1 out]
      }
      frame "Save" {
        n333 = Unbundle By Name(w753) -> ("Config Saved"=w743:T9, "Config Path"=w742:path, "Config"=w751:T9, "Channel Display"=w750:T7, "Changes?"=w739:bool)
        n334 = call "Store Channel Display.vi"("Channels in"=w751, "Channel Display"=w750) -> ("Channels out"=w744:T9)  [unwired: 13 in]
        n335 = Flatten To String(anything=w744) -> (data string=w756:string)  [unwired: 3 in, 2 out]
        n336 = call "Write Characters To File with Advisory Dialog Option and Error Out.vi"("file path (dialog if empty)"=w742, "character string"=w756, "advisory dialog? (display:T)"=FALSE, "pattern"="*.cfg") -> ("new file path (Not A Path if cancelled)"=w754:path, "error out"=w755:errorcluster)  [unwired: 10 in]
        n337 = case shown="No Error" w755 {
          tunnel: w754 -> [w760 _]
          tunnel: [w760 w764] -> w749
          tunnel: w742 -> [_ w764]
          tunnel: [w761 w763] -> w745
          tunnel: w744 -> [w761 _]
          tunnel: w743 -> [_ w763]
          tunnel: [FALSE ("Changes?") w762] -> w740
          tunnel: w739 -> [w757 w762]
          tunnel: [w757 w762] -> w738
          frame No Error {
            w758 = T21."Disabled and Grayed Out" ("Disabled")
            n338 = property on="Save" class="Bool"("DisabledEnum"=w758) -> ()  [unwired: 2 in, 2 out]
            n339 = property on="Revert" class="Bool"("DisabledEnum"=w758) -> ()  [unwired: 2 in, 2 out]
          }
          frame Error {
          }
        }
        "Changes Latch" <- w738
        n340 = Current VI's Path() -> (path=w748:path)
        n341 = Bundle By Name(cluster=w753, "Config Saved"=w745, "Config Path"=w749, "Changes?"=w740) -> (w752:T19)
        n342 = call "Insert Multiple Events.vi"("Events to Insert"=string[] ["Remember Config"], "Event queue in"=w735) -> ("Event queue out"=w736:string[])  [unwired: 5 in]
        n343 = call "Set Window Title using Path.vi"("VI path"=w748, "File Path"=w749, "Title"="Sensor Configuration") -> ()  [unwired: 12 in, 1 out]
      }
      frame "Remember Config" {
        # "Save last config path to ini."
        n344 = Unbundle By Name(w773) -> ("Config Path"=w769:path, "App Config Path"=w766:path)
        n345 = call <vilib>:"Open Config Data.vi"("configuration file path"=w766) -> ("error out"=w772:errorcluster, "refnum"=w771:T27)  [unwired: 8 in, 1 out]
        n346 = call-poly <vilib>:"Write Key.vi"("section"="App Config", "error in (no error)"=w772, "value"=w769, "key"="Last Config", "refnum"=w771) -> ("error out"=w768:errorcluster, "refnum out"=w767:T27)  [unwired: 4 in, 1 out]
        n347 = call <vilib>:"Close Config Data.vi"("error in (no error)"=w768, "refnum"=w767) -> ()  [unwired: 8 in, 2 out]
      }
      frame "Clear" {
        w776 = T21."Disabled and Grayed Out" ("Disabled")
        w778 = string[][] [] ("Header Table")
        n348 = local write "Config Name"("" ("Config Name")) -> ()
        n349 = property on="Save" class="Bool"("DisabledEnum"=w776) -> ()  [unwired: 2 in, 2 out]
        n350 = property on="Revert" class="Bool"("DisabledEnum"=w776) -> ()  [unwired: 2 in, 2 out]
        n351 = local write "Header Table"(w778) -> ()
        n352 = local write "DAQ Table"(w778) -> ()
        n353 = Bundle By Name(cluster=w785, "Config Path"=path "" ("Sensor Config Path"), "Config"=T9 {"DAQ Settings"={"Trigger Type"=enum."Manual", "Trigger Samples"=0, "Pretrigger Samples"=0, "Trigger Interval"=0.0, "Time Units"=FALSE, "Auto Save"=FALSE, "Sample Rate"=0.0, "Select Analog"=FALSE, "Trigger Value"=0.0, "Trigger Stop Method"=enum."Use Samples Value to Stop Trigger", "Rate Sec/Min"=FALSE, "Save Mode"=enum."Single File", "File Size Limit"=0.0, "Log File Type"=enum."Basic", "Trigger Data Index"=0}, "Channels"=[], "Header"={"TA Number"="", "Test Name"="", "Serial Number"="", "Technician"=""}, "Graph Settings"={"Graph Labels"=[], [], [], [], [], [], [], [], [], [], [], [], [], "Graph Toggles"=[], "Axis Toggles"=[], "Graph Range"=enum."1"}, "Test Limits"=[], "All Type Info"=[], "Save Mode"=enum."New File at Midnight"}) -> (w784:T19)
        n354 = call "Insert Single Event.vi"("Insert?"=TRUE, "Event to insert"="Init", "Event queue in"=w782) -> ("Event queue out"=w783:string[])  [unwired: 4 in]
      }
      frame "Update DAQ Table" {
        w802 = i16 3 ("precision (6)")
        w804 = ""
        n355 = Unbundle By Name(w822) -> ("Config.DAQ Settings.Log File Type"=w793:T3, "Config.DAQ Settings.Trigger Type"=w818:T6, "Config.DAQ Settings.Time Units"=w815:bool, "Config.DAQ Settings.Rate Sec/Min"=w800:bool, "Config.DAQ Settings.Auto Save"=w814:bool, "Config.DAQ Settings.Trigger Stop Method"=w817:T11, "Config.DAQ Settings.Save Mode"=w795:T4, "Config.DAQ Settings.File Size Limit"=w794:dbl, "Config.DAQ Settings.Trigger Value"=w813:dbl, "Config.DAQ Settings.Trigger Samples"=w811:i32, "Config.DAQ Settings.Pretrigger Samples"=w809:i32, "Config.DAQ Settings.Trigger Interval"=w807:dbl, "Config.DAQ Settings.Sample Rate"=w805:dbl, "Config.Channels"=w792:T12[], "Config.DAQ Settings.Trigger Data Index"=w791:u32)
        n356 = Index Array(array=w792, index=w791) -> (element=w790:T12)
        n357 = Unbundle By Name(w790) -> ("Channel"=w788:string, "Name"=w787:string)
        n358 = Empty String/Path?(string/path=w787) -> (empty?=w789:bool)
        n359 = Select(t=w788, s=w789, f=w787) -> (s? t:f=w786:string)
        n360 = Number To Fractional String(number=w813, precision (6)=w802) -> (F-format string=w812:string)  [unwired: 2 in]
        n361 = Number To Decimal String(number=w811) -> (decimal integer string=w810:string)  [unwired: 1 in]
        n362 = Number To Decimal String(number=w809) -> (decimal integer string=w808:string)  [unwired: 1 in]
        n363 = Number To Fractional String(number=w807, precision (6)=w802) -> (F-format string=w806:string)  [unwired: 2 in]
        n364 = Number To Decimal String(number=w805) -> (decimal integer string=w803:string)  [unwired: 1 in]
        n365 = Not(x=w800) -> (.not. x?=w801:bool)
        n366 = Not(x=w815) -> (.not. x?=w816:bool)
        n367 = Build Array(w804, w786, w812, w810, w808, w806, w804, w803) -> (w821:string[])
        n368 = local write "Log File Type"(w793) -> ()
        n369 = local write "Trigger Type"(w818) -> ()
        n370 = local write "Hours"(w815) -> ()
        n371 = local write "Minutes"(w816) -> ()
        n372 = local write "Sample Min"(w800) -> ()
        n373 = local write "Sample Sec"(w801) -> ()
        n374 = local write "Auto Save"(w814) -> ()
        n375 = local write "Trigger Stop Method"(w817) -> ()
        n376 = local write "Save Mode"(w795) -> ()
        n377 = local write "Limit:"(w794) -> ()
        n378 = Build Array(w821) -> (w820:string[][])
        n379 = Transpose 2D Array(2D array=w820) -> (transposed array=w819:string[][])
        n380 = local write "DAQ Table"(w819) -> ()
        n381 = call "Insert Single Event.vi"("Insert?"=TRUE, "Event to insert"="Update Fields", "Event queue in"=w796) -> ("Event queue out"=w797:string[])  [unwired: 4 in]
      }
      frame "Update Fields" {
        n382 = Unbundle By Name(w832) -> ("Config.DAQ Settings.Trigger Type"=w831:T6, "Config.DAQ Settings.Save Mode"=w824:T4)
        n383 = case shown="\"Single File\", \"New File at Midnight\", Default" w824 {
          tunnel: [FALSE TRUE] -> w823
          frame "Single File", "New File at Midnight", Default {
          }
          frame "Segmented Files" {
          }
        }
        n384 = case shown="\"Timed\"" w831 {
          tunnel: [w836 w838 w840] -> w830
          tunnel: [w836 w838 w840] -> w829
          tunnel: [w836 w837 w840] -> w828
          tunnel: [w836 w838 w840] -> w827
          tunnel: [w836 w837 TRUE] -> w826
          tunnel: [w836 w838 w840] -> w825
          frame "Manual", Default {
            w836 = TRUE
          }
          frame "Timed" {
            w837 = FALSE
            w838 = TRUE
          }
          frame "Analog Rising", "Analog Falling" {
            w840 = FALSE
          }
        }
        n385 = property on="Hide Trig Ch" class="Bool"("Visible"=w830) -> ()  [unwired: 2 in, 2 out]
        n386 = property on="Hide Trig Val" class="Bool"("Visible"=w829) -> ()  [unwired: 2 in, 2 out]
        n387 = property on="Hide Trig Samples" class="Bool"("Visible"=w828) -> ()  [unwired: 2 in, 2 out]
        n388 = property on="Hide Pretrig Smpls" class="Bool"("Visible"=w827) -> ()  [unwired: 2 in, 2 out]
        n389 = property on="Hide Trig Int" class="Bool"("Visible"=w826) -> ()  [unwired: 2 in, 2 out]
        n390 = property on="Hide Trig Stop" class="Bool"("Visible"=w825) -> ()  [unwired: 2 in, 2 out]
        n391 = property on="Limit:" class="DigNum (strict)"("Visible"=w823) -> ()  [unwired: 2 in, 2 out]
      }
    }
  }
